vi "DetectorTest_MainV2.vi"() -> ()   [LabVIEW 2012]
uses:
  <vilib>/Analysis/NI_AALBase.lvlib
panel:
  out "Counter":i32
  out "NameList":string[](array[string])=["Diode_Open_3000", "Diode_Open_2000", "Diode_Open_1000", "Diode_Open_500", "Diode_Open_300", "Diode_Open_200", "Diode_Open_100", "Diode_Open_70", "Diode_Open_50", "Diode_Open_20", "Diode_Open_5_500", "Diode_Open_5_300", "Diode_Open_5_200", "Diode_Open_5_100", "Diode_Open_5_70", "Diode_Open_5_50", "Diode_Open_5_20", "Diode_Full_500", "Diode_Full_300", "Diode_Full_200", "Diode_Full_100", "Diode_Full_70", "Diode_Full_50", "Diode_Full_20", "Diode_Open_100_A", "Diode_Open_200_A", "QE_pad"]
  in  "Wafer Info Flash 2":T1={"Cell Name"="5500_130_05", "Package"="", "Coating"="", "LRC?"=enum."J2", "Comment"=""}
  in  "Parameters Flash 2":T2 {"Voc" format="%#_4g"; "Isc" format="%#_4g"; "FF" format="%#_4g"; "Imax" format="%#_4g"; "Vmax" format="%#_4g"; "Pmax" format="%#_4g"; "Itest" format="%#_4g"}
  in  "Wafer Info Flash":T1={"Cell Name"="Diode_Open_5_100", "Package"="", "Coating"="", "LRC?"=enum."J2", "Comment"=""}
  in  "Parameters Flash":T2={"Voc"=0.0, "Isc"=0.0, "FF"=0.0, "Vtest"=0.0, "Imax"=0.0, "Vmax"=0.0, "Pmax"=0.0, "Itest"=0.0, "Efficiency"=0.0, "P_in (W)"=0.0, "Irradiance (W/cm²)"=0.0, "Cell Area (cm²)"=12801.99006, "Number of AM1.5D Suns"=0.0, "Isotype Scalar"=0.0, "Equivalent 1 sun Jsc"=0.0} {"Voc" format="%#_4g"; "Isc" format="%#_4g"; "FF" format="%#_4g"; "Imax" format="%#_4g"; "Vmax" format="%#_4g"; "Pmax" format="%#_4g"; "Itest" format="%#_4g"}
  out "RawData file":path=path "C:/Users/Flash/Desktop/Data/Detector test data/A-3348-2-A_Diode_Open_5_100_20171205171726.csv"
  out "Fine Cell Clusters":T3(array[cluster])=[{"Cell Name"="Diode_Open_5_100", "X-coord"=56060.0, "Y-coord"=24330.0, "Area"=12801.99006, "Grid Shadowing"=0.0, "Xdim"=50.0, "Ydim"=50.0, "Mesa Area"=7853.981634}, {"Cell Name"="Diode_Open_5_100", "X-coord"=56060.0, "Y-coord"=14330.0, "Area"=12801.99006, "Grid Shadowing"=0.0, "Xdim"=50.0, "Ydim"=50.0, "Mesa Area"=7853.981634}, {"Cell Name"="Diode_Open_5_100", "X-coord"=-3940.0, "Y-coord"=4330.0, "Area"=12801.99006, "Grid Shadowing"=0.0, "Xdim"=50.0, "Ydim"=50.0, "Mesa Area"=7853.981634}, {"Cell Name"="Diode_Open_5_100", "X-coord"=-9540.0, "Y-coord"=10700.0, "Area"=12801.99006, "Grid Shadowing"=0.0, "Xdim"=50.0, "Ydim"=50.0, "Mesa Area"=7853.981634}, {"Cell Name"="Diode_Open_5_100", "X-coord"=46060.0, "Y-coord"=4330.0, "Area"=12801.99006, "Grid Shadowing"=0.0, "Xdim"=50.0, "Ydim"=50.0, "Mesa Area"=7853.981634}, {"Cell Name"="Diode_Open_5_100", "X-coord"=6060.0, "Y-coord"=-5670.0, "Area"=12801.99006, "Grid Shadowing"=0.0, "Xdim"=50.0, "Ydim"=50.0, "Mesa Area"=7853.981634}, {"Cell Name"="Diode_Open_5_100", "X-coord"=460.0, "Y-coord"=700.0, "Area"=12801.99006, "Grid Shadowing"=0.0, "Xdim"=50.0, "Ydim"=50.0, "Mesa Area"=7853.981634}, {"Cell Name"="Diode_Open_5_100", "X-coord"=16060.0, "Y-coord"=-5670.0, "Area"=12801.99006, "Grid Shadowing"=0.0, "Xdim"=50.0, "Ydim"=50.0, "Mesa Area"=7853.981634}, {"Cell Name"="Diode_Open_5_100", "X-coord"=26060.0, "Y-coord"=-5670.0, "Area"=12801.99006, "Grid Shadowing"=0.0, "Xdim"=50.0, "Ydim"=50.0, "Mesa Area"=7853.981634}, {"Cell Name"="Diode_Open_5_100", "X-coord"=30460.0, "Y-coord"=700.0, "Area"=12801.99006, "Grid Shadowing"=0.0, "Xdim"=50.0, "Ydim"=50.0, "Mesa Area"=7853.981634}]
  out "Selected Data":cluster{dbl[], dbl[]}={[nan, nan, nan, nan, nan, nan, nan, nan, nan, nan, nan, nan, nan, nan, nan, nan, nan, nan, nan, nan, nan, nan, nan, nan, nan, nan, nan, nan, nan, nan, nan, nan, nan, nan, nan, nan, nan, nan, nan, nan, nan, nan, nan, nan, nan, nan, nan, nan, nan, nan, nan, nan, nan, nan, nan, nan, nan, nan, nan, nan, nan, nan, nan, nan, nan, nan, nan, nan, nan, nan, nan, nan, nan, nan, nan, nan, nan, nan, nan, nan, nan, nan, nan, nan, nan, nan, nan, nan, nan, nan, nan, nan, nan, nan, nan, nan, nan, nan, nan, nan, nan, nan, nan, nan], [nan, nan, nan, nan, nan, nan, nan, nan, nan, nan, nan, nan, nan, nan, nan, nan, nan, nan, nan, nan, nan, nan, nan, nan, nan, nan, nan, nan, nan, nan, nan, nan, nan, nan, nan, nan, nan, nan, nan, nan, nan, nan, nan, nan, nan, nan, nan, nan, nan, nan, nan, nan, nan, nan, nan, nan, nan, nan, nan, nan, nan, nan, nan, nan, nan, nan, nan, nan, nan, nan, nan, nan, nan, nan, nan, nan, nan, nan, nan, nan, nan, nan, nan, nan, nan, nan, nan, nan, nan, nan, nan, nan, nan, nan, nan, nan, nan, nan, nan, nan, nan, nan, nan, nan]}
  in  "Test Results 2":T4
  in  "Session Info 2":T5={"V set"=-1.0, "I compliance"=0.001, "J set"=0.01, "I set"=0.0, "V compliance"=1.0, "Laser Power (mW)"=0.0, "TestID"=0, "Session Time"=timestamp(0 s since 1904-01-01), "Operator"="Radek"} {"V compliance" format="%#_6f"; "I compliance" format="%#_6e"}
  in  "Die Info 2":T6={"Device Name"="", "ActiveArea_um2"=3848.451, "MesaArea_um2"=3848.451, "x"=0.0, "y"=0.0}
  in  "Wafer Info 2":T7
  in  "Test Results":T4={"I meas"=-8.21153e-09, "V meas"=0.229564, "Time"=timestamp(3595368212.7604895 s since 1904-01-01)}
  in  "Session Info":T5={"V set"=-1.0, "I compliance"=0.001, "J set"=0.01, "I set"=1.5393804e-06, "V compliance"=1.0, "Laser Power (mW)"=0.0, "TestID"=289, "Session Time"=timestamp(3595367846.336531 s since 1904-01-01), "Operator"="pkawula"} {"V compliance" format="%#_6f"; "I compliance" format="%#_6e"}
  in  "Die Info":T6={"Device Name"="Diode_Open_5_100", "ActiveArea_um2"=12801.99006, "MesaArea_um2"=7853.981634, "x"=6060.0, "y"=44330.0}
  in  "Wafer Info":T7={"Wafer Name"="A-3348-2-A", "Scribe"="BG531-103", "Mask"="SL066", "Lot"="SJC_ENG_342_4"}
  in  "Name Array":string[](array[string])=["Wafer name", "Scribe", "Mask", "Lot", "Device name", "Active Area", "Mesa Area", "x", "y", "Imeas", "Vmeas", "Time", "Vset", "Icomp", "Jset", "Iset", "Vcomp", "Laser Power", "TestID", "SessionTime", "Operator", "Selected"]
  in  "TestID file":path=path "C:/Users/Flash/Desktop/LabVIEW/Detector IV/rawtest_log.csv"
  in  "update wafer":bool
  in  "Lot":string="SJC_ENG_342_4"
  in  "Laser Power (mW)":dbl
  in  "Device Name":string="Diode_Open_5_100"
  in  "Scribe":string="BG531-105"
  in  "MesaArea_um2":dbl=7853.981634
  out "Status":string="idle"
  out "error out":errorcluster
  in  "error in (no error)":errorcluster
  out "Manaul Plot 1":cluster{"V manual":dbl[], dbl[]}[](array[cluster])=[{"V manual"=[-1.5, -1.45128, -1.40256, -1.35385, -1.30513, -1.25641, -1.20769, -1.15897, -1.11026, -1.06154, -1.01282, -0.964103, -0.915385, -0.866667, -0.817949, -0.769231, -0.720513, -0.671795, -0.623077, -0.574359, -0.525641, -0.476923, -0.428205, -0.379487, -0.330769, -0.282051, -0.233333, -0.184615, -0.135897, -0.0871795, -0.0384615, 0.0102564, 0.0589744, 0.107692, 0.15641, 0.205128, 0.253846, 0.302564, 0.351282, 0.4], [0.000371182, 0.000368087, 0.000365666, 0.000361585, 0.000358777, 0.000355415, 0.000352273, 0.00034839, 0.000345122, 0.00034151, 0.00033751, 0.000332836, 0.000329855, 0.000326461, 0.000322528, 0.000317656, 0.000313266, 0.000310053, 0.000304697, 0.000300113, 0.00029575, 0.000290713, 0.000285749, 0.00028048, 0.000275303, 0.000269023, 0.000263057, 0.000256756, 0.000250067, 0.000242646, 0.000235352, 0.000226249, 0.000216807, 0.000205541, 0.000192231, 0.000174354, 0.000146988, 9.49448e-05, 1.32493e-05, 0.000227531]}, {"V manual"=[-1.0, nan, nan, nan, nan, nan, nan, nan, nan, nan, nan, nan, nan, nan, nan, nan, nan, nan, nan, nan, nan, nan, nan, nan, nan, nan, nan, nan, nan, nan, nan, nan, nan, nan, nan, nan, nan, nan, nan, nan], [0.0003364616, nan, nan, nan, nan, nan, nan, nan, nan, nan, nan, nan, nan, nan, nan, nan, nan, nan, nan, nan, nan, nan, nan, nan, nan, nan, nan, nan, nan, nan, nan, nan, nan, nan, nan, nan, nan, nan, nan, nan]}, {"V manual"=[0.369974, nan, nan, nan, nan, nan, nan, nan, nan, nan, nan, nan, nan, nan, nan, nan, nan, nan, nan, nan, nan, nan, nan, nan, nan, nan, nan, nan, nan, nan, nan, nan, nan, nan, nan, nan, nan, nan, nan, nan], [8.183848863e-05, nan, nan, nan, nan, nan, nan, nan, nan, nan, nan, nan, nan, nan, nan, nan, nan, nan, nan, nan, nan, nan, nan, nan, nan, nan, nan, nan, nan, nan, nan, nan, nan, nan, nan, nan, nan, nan, nan, nan]}]
  out "Manual Plot 0":cluster{"V manual":dbl[], "I manual":dbl[]}[](array[cluster])=[{"V manual"=[-1.5, -1.45128, -1.40256, -1.35385, -1.30513, -1.25641, -1.20769, -1.15897, -1.11026, -1.06154, -1.01282, -0.964103, -0.915385, -0.866667, -0.817949, -0.769231, -0.720513, -0.671795, -0.623077, -0.574359, -0.525641, -0.476923, -0.428205, -0.379487, -0.330769, -0.282051, -0.233333, -0.184615, -0.135897, -0.0871795, -0.0384615, 0.0102564, 0.0589744, 0.107692, 0.15641, 0.205128, 0.253846, 0.302564, 0.351282, 0.4], "I manual"=[-0.000371182, -0.000368087, -0.000365666, -0.000361585, -0.000358777, -0.000355415, -0.000352273, -0.00034839, -0.000345122, -0.00034151, -0.00033751, -0.000332836, -0.000329855, -0.000326461, -0.000322528, -0.000317656, -0.000313266, -0.000310053, -0.000304697, -0.000300113, -0.00029575, -0.000290713, -0.000285749, -0.00028048, -0.000275303, -0.000269023, -0.000263057, -0.000256756, -0.000250067, -0.000242646, -0.000235352, -0.000226249, -0.000216807, -0.000205541, -0.000192231, -0.000174354, -0.000146988, -9.49448e-05, 1.32493e-05, 0.000227531]}, {"V manual"=[-1.0, nan, nan, nan, nan, nan, nan, nan, nan, nan, nan, nan, nan, nan, nan, nan, nan, nan, nan, nan, nan, nan, nan, nan, nan, nan, nan, nan, nan, nan, nan, nan, nan, nan, nan, nan, nan, nan, nan, nan], "I manual"=[-0.0003364616, nan, nan, nan, nan, nan, nan, nan, nan, nan, nan, nan, nan, nan, nan, nan, nan, nan, nan, nan, nan, nan, nan, nan, nan, nan, nan, nan, nan, nan, nan, nan, nan, nan, nan, nan, nan, nan, nan, nan]}, {"V manual"=[0.369974, nan, nan, nan, nan, nan, nan, nan, nan, nan, nan, nan, nan, nan, nan, nan, nan, nan, nan, nan, nan, nan, nan, nan, nan, nan, nan, nan, nan, nan, nan, nan, nan, nan, nan, nan, nan, nan, nan, nan], "I manual"=[8.183848863e-05, nan, nan, nan, nan, nan, nan, nan, nan, nan, nan, nan, nan, nan, nan, nan, nan, nan, nan, nan, nan, nan, nan, nan, nan, nan, nan, nan, nan, nan, nan, nan, nan, nan, nan, nan, nan, nan, nan, nan]}]
  in  "Reset 1st die":bool
  in  "Sweep Settings":T8={"Channel"=enum."Channel A", "Vstart"=-2.0, "Vend"=0.5, "# of points"=30, "NPLC"=1.0, "I compliance"=0.001, "Delay ms"=500.0}
  in  "Reset xy":bool
  out "current y":i32
  out "current x":i32
  in  "sweep delay ms":dbl=500.0
  in  "I compliance":dbl=0.001
  in  "points":u16=40
  in  "V end":dbl=0.4
  in  "V start":dbl=-1.5
  in  "Repeat Vf":u32=1
  out "I set":dbl=7.853981633999999e-07
  in  "V compliance":dbl=1.0 format="%#_6f"
  in  "Vf delay ms":dbl=100.0
  in  "J set A/cm2":dbl=0.01
  in  "Repeat Id":u32=5
  in  "I compliance":dbl=0.001 format="%#_6e"
  in  "Id delay ms":dbl=500.0
  in  "V set":dbl=-1.0
  out "Vmeas Settings":T9={"Channel"=enum."Channel A", "Iset"=-1.0, "NPLC"=1.0, "V compliance"=0.001, "Repeat time"=3, "Delay ms"=500.0}
  out "Imeas Settings":T10={"Channel"=enum."Channel A", "Vset"=-1.0, "NPLC"=1.0, "I compliance"=0.001, "Repeat time"=3, "Delay ms"=500.0}
  out "Array of Cell Data Clusters":T11(array[cluster])=[{"Cell Name"="Diode_Open_5_100", "X-coord"=-13940.0, "Y-coord"=24330.0, "Area"=12801.99006, "Grid Shadowing"=0.0, "Ydim"=50.0, "Xdim"=50.0, "Meas Area"=7853.981634}, {"Cell Name"="Diode_Open_5_100", "X-coord"=-19540.0, "Y-coord"=30700.0, "Area"=12801.99006, "Grid Shadowing"=0.0, "Ydim"=50.0, "Xdim"=50.0, "Meas Area"=7853.981634}, {"Cell Name"="Diode_Open_5_100", "X-coord"=-3940.0, "Y-coord"=24330.0, "Area"=12801.99006, "Grid Shadowing"=0.0, "Ydim"=50.0, "Xdim"=50.0, "Meas Area"=7853.981634}, {"Cell Name"="Diode_Open_5_100", "X-coord"=-9540.0, "Y-coord"=30700.0, "Area"=12801.99006, "Grid Shadowing"=0.0, "Ydim"=50.0, "Xdim"=50.0, "Meas Area"=7853.981634}, {"Cell Name"="Diode_Open_5_100", "X-coord"=6060.0, "Y-coord"=24330.0, "Area"=12801.99006, "Grid Shadowing"=0.0, "Ydim"=50.0, "Xdim"=50.0, "Meas Area"=7853.981634}, {"Cell Name"="Diode_Open_5_100", "X-coord"=460.0, "Y-coord"=30700.0, "Area"=12801.99006, "Grid Shadowing"=0.0, "Ydim"=50.0, "Xdim"=50.0, "Meas Area"=7853.981634}, {"Cell Name"="Diode_Open_5_100", "X-coord"=16060.0, "Y-coord"=24330.0, "Area"=12801.99006, "Grid Shadowing"=0.0, "Ydim"=50.0, "Xdim"=50.0, "Meas Area"=7853.981634}, {"Cell Name"="Diode_Open_5_100", "X-coord"=10460.0, "Y-coord"=30700.0, "Area"=12801.99006, "Grid Shadowing"=0.0, "Ydim"=50.0, "Xdim"=50.0, "Meas Area"=7853.981634}, {"Cell Name"="Diode_Open_5_100", "X-coord"=26060.0, "Y-coord"=24330.0, "Area"=12801.99006, "Grid Shadowing"=0.0, "Ydim"=50.0, "Xdim"=50.0, "Meas Area"=7853.981634}, {"Cell Name"="Diode_Open_5_100", "X-coord"=20460.0, "Y-coord"=30700.0, "Area"=12801.99006, "Grid Shadowing"=0.0, "Ydim"=50.0, "Xdim"=50.0, "Meas Area"=7853.981634}, {"Cell Name"="Diode_Open_5_100", "X-coord"=36060.0, "Y-coord"=24330.0, "Area"=12801.99006, "Grid Shadowing"=0.0, "Ydim"=50.0, "Xdim"=50.0, "Meas Area"=7853.981634}, {"Cell Name"="Diode_Open_5_100", "X-coord"=30460.0, "Y-coord"=30700.0, "Area"=12801.99006, "Grid Shadowing"=0.0, "Ydim"=50.0, "Xdim"=50.0, "Meas Area"=7853.981634}, {"Cell Name"="Diode_Open_5_100", "X-coord"=46060.0, "Y-coord"=24330.0, "Area"=12801.99006, "Grid Shadowing"=0.0, "Ydim"=50.0, "Xdim"=50.0, "Meas Area"=7853.981634}, {"Cell Name"="Diode_Open_5_100", "X-coord"=40460.0, "Y-coord"=30700.0, "Area"=12801.99006, "Grid Shadowing"=0.0, "Ydim"=50.0, "Xdim"=50.0, "Meas Area"=7853.981634}, {"Cell Name"="Diode_Open_5_100", "X-coord"=56060.0, "Y-coord"=24330.0, "Area"=12801.99006, "Grid Shadowing"=0.0, "Ydim"=50.0, "Xdim"=50.0, "Meas Area"=7853.981634}, {"Cell Name"="Diode_Open_5_100", "X-coord"=50460.0, "Y-coord"=30700.0, "Area"=12801.99006, "Grid Shadowing"=0.0, "Ydim"=50.0, "Xdim"=50.0, "Meas Area"=7853.981634}, {"Cell Name"="Diode_Open_5_100", "X-coord"=-13940.0, "Y-coord"=14330.0, "Area"=12801.99006, "Grid Shadowing"=0.0, "Ydim"=50.0, "Xdim"=50.0, "Meas Area"=7853.981634}, {"Cell Name"="Diode_Open_5_100", "X-coord"=-19540.0, "Y-coord"=20700.0, "Area"=12801.99006, "Grid Shadowing"=0.0, "Ydim"=50.0, "Xdim"=50.0, "Meas Area"=7853.981634}, {"Cell Name"="Diode_Open_5_100", "X-coord"=-3940.0, "Y-coord"=14330.0, "Area"=12801.99006, "Grid Shadowing"=0.0, "Ydim"=50.0, "Xdim"=50.0, "Meas Area"=7853.981634}, {"Cell Name"="Diode_Open_5_100", "X-coord"=-9540.0, "Y-coord"=20700.0, "Area"=12801.99006, "Grid Shadowing"=0.0, "Ydim"=50.0, "Xdim"=50.0, "Meas Area"=7853.981634}, {"Cell Name"="Diode_Open_5_100", "X-coord"=16060.0, "Y-coord"=14330.0, "Area"=12801.99006, "Grid Shadowing"=0.0, "Ydim"=50.0, "Xdim"=50.0, "Meas Area"=7853.981634}, {"Cell Name"="Diode_Open_5_100", "X-coord"=10460.0, "Y-coord"=20700.0, "Area"=12801.99006, "Grid Shadowing"=0.0, "Ydim"=50.0, "Xdim"=50.0, "Meas Area"=7853.981634}, {"Cell Name"="Diode_Open_5_100", "X-coord"=26060.0, "Y-coord"=14330.0, "Area"=12801.99006, "Grid Shadowing"=0.0, "Ydim"=50.0, "Xdim"=50.0, "Meas Area"=7853.981634}, {"Cell Name"="Diode_Open_5_100", "X-coord"=20460.0, "Y-coord"=20700.0, "Area"=12801.99006, "Grid Shadowing"=0.0, "Ydim"=50.0, "Xdim"=50.0, "Meas Area"=7853.981634}, {"Cell Name"="Diode_Open_5_100", "X-coord"=46060.0, "Y-coord"=14330.0, "Area"=12801.99006, "Grid Shadowing"=0.0, "Ydim"=50.0, "Xdim"=50.0, "Meas Area"=7853.981634}, {"Cell Name"="Diode_Open_5_100", "X-coord"=40460.0, "Y-coord"=20700.0, "Area"=12801.99006, "Grid Shadowing"=0.0, "Ydim"=50.0, "Xdim"=50.0, "Meas Area"=7853.981634}, {"Cell Name"="Diode_Open_5_100", "X-coord"=56060.0, "Y-coord"=14330.0, "Area"=12801.99006, "Grid Shadowing"=0.0, "Ydim"=50.0, "Xdim"=50.0, "Meas Area"=7853.981634}, {"Cell Name"="Diode_Open_5_100", "X-coord"=50460.0, "Y-coord"=20700.0, "Area"=12801.99006, "Grid Shadowing"=0.0, "Ydim"=50.0, "Xdim"=50.0, "Meas Area"=7853.981634}, {"Cell Name"="Diode_Open_5_100", "X-coord"=-3940.0, "Y-coord"=4330.0, "Area"=12801.99006, "Grid Shadowing"=0.0, "Ydim"=50.0, "Xdim"=50.0, "Meas Area"=7853.981634}, {"Cell Name"="Diode_Open_5_100", "X-coord"=-9540.0, "Y-coord"=10700.0, "Area"=12801.99006, "Grid Shadowing"=0.0, "Ydim"=50.0, "Xdim"=50.0, "Meas Area"=7853.981634}, {"Cell Name"="Diode_Open_5_100", "X-coord"=6060.0, "Y-coord"=4330.0, "Area"=12801.99006, "Grid Shadowing"=0.0, "Ydim"=50.0, "Xdim"=50.0, "Meas Area"=7853.981634}, {"Cell Name"="Diode_Open_5_100", "X-coord"=460.0, "Y-coord"=10700.0, "Area"=12801.99006, "Grid Shadowing"=0.0, "Ydim"=50.0, "Xdim"=50.0, "Meas Area"=7853.981634}, {"Cell Name"="Diode_Open_5_100", "X-coord"=16060.0, "Y-coord"=4330.0, "Area"=12801.99006, "Grid Shadowing"=0.0, "Ydim"=50.0, "Xdim"=50.0, "Meas Area"=7853.981634}, {"Cell Name"="Diode_Open_5_100", "X-coord"=10460.0, "Y-coord"=10700.0, "Area"=12801.99006, "Grid Shadowing"=0.0, "Ydim"=50.0, "Xdim"=50.0, "Meas Area"=7853.981634}, {"Cell Name"="Diode_Open_5_100", "X-coord"=26060.0, "Y-coord"=4330.0, "Area"=12801.99006, "Grid Shadowing"=0.0, "Ydim"=50.0, "Xdim"=50.0, "Meas Area"=7853.981634}, {"Cell Name"="Diode_Open_5_100", "X-coord"=20460.0, "Y-coord"=10700.0, "Area"=12801.99006, "Grid Shadowing"=0.0, "Ydim"=50.0, "Xdim"=50.0, "Meas Area"=7853.981634}, {"Cell Name"="Diode_Open_5_100", "X-coord"=36060.0, "Y-coord"=4330.0, "Area"=12801.99006, "Grid Shadowing"=0.0, "Ydim"=50.0, "Xdim"=50.0, "Meas Area"=7853.981634}, {"Cell Name"="Diode_Open_5_100", "X-coord"=30460.0, "Y-coord"=10700.0, "Area"=12801.99006, "Grid Shadowing"=0.0, "Ydim"=50.0, "Xdim"=50.0, "Meas Area"=7853.981634}, {"Cell Name"="Diode_Open_5_100", "X-coord"=46060.0, "Y-coord"=4330.0, "Area"=12801.99006, "Grid Shadowing"=0.0, "Ydim"=50.0, "Xdim"=50.0, "Meas Area"=7853.981634}, {"Cell Name"="Diode_Open_5_100", "X-coord"=40460.0, "Y-coord"=10700.0, "Area"=12801.99006, "Grid Shadowing"=0.0, "Ydim"=50.0, "Xdim"=50.0, "Meas Area"=7853.981634}, {"Cell Name"="Diode_Open_5_100", "X-coord"=6060.0, "Y-coord"=-5670.0, "Area"=12801.99006, "Grid Shadowing"=0.0, "Ydim"=50.0, "Xdim"=50.0, "Meas Area"=7853.981634}, {"Cell Name"="Diode_Open_5_100", "X-coord"=460.0, "Y-coord"=700.0, "Area"=12801.99006, "Grid Shadowing"=0.0, "Ydim"=50.0, "Xdim"=50.0, "Meas Area"=7853.981634}, {"Cell Name"="Diode_Open_5_100", "X-coord"=16060.0, "Y-coord"=-5670.0, "Area"=12801.99006, "Grid Shadowing"=0.0, "Ydim"=50.0, "Xdim"=50.0, "Meas Area"=7853.981634}, {"Cell Name"="Diode_Open_5_100", "X-coord"=10460.0, "Y-coord"=700.0, "Area"=12801.99006, "Grid Shadowing"=0.0, "Ydim"=50.0, "Xdim"=50.0, "Meas Area"=7853.981634}, {"Cell Name"="Diode_Open_5_100", "X-coord"=26060.0, "Y-coord"=-5670.0, "Area"=12801.99006, "Grid Shadowing"=0.0, "Ydim"=50.0, "Xdim"=50.0, "Meas Area"=7853.981634}, {"Cell Name"="Diode_Open_5_100", "X-coord"=20460.0, "Y-coord"=700.0, "Area"=12801.99006, "Grid Shadowing"=0.0, "Ydim"=50.0, "Xdim"=50.0, "Meas Area"=7853.981634}, {"Cell Name"="Diode_Open_5_100", "X-coord"=36060.0, "Y-coord"=-5670.0, "Area"=12801.99006, "Grid Shadowing"=0.0, "Ydim"=50.0, "Xdim"=50.0, "Meas Area"=7853.981634}, {"Cell Name"="Diode_Open_5_100", "X-coord"=30460.0, "Y-coord"=700.0, "Area"=12801.99006, "Grid Shadowing"=0.0, "Ydim"=50.0, "Xdim"=50.0, "Meas Area"=7853.981634}, {"Cell Name"="Diode_Open_5_100", "X-coord"=6060.0, "Y-coord"=54330.0, "Area"=12801.99006, "Grid Shadowing"=0.0, "Ydim"=50.0, "Xdim"=50.0, "Meas Area"=7853.981634}, {"Cell Name"="Diode_Open_5_100", "X-coord"=460.0, "Y-coord"=60700.0, "Area"=12801.99006, "Grid Shadowing"=0.0, "Ydim"=50.0, "Xdim"=50.0, "Meas Area"=7853.981634}, {"Cell Name"="Diode_Open_5_100", "X-coord"=6060.0, "Y-coord"=64330.0, "Area"=12801.99006, "Grid Shadowing"=0.0, "Ydim"=50.0, "Xdim"=50.0, "Meas Area"=7853.981634}, {"Cell Name"="Diode_Open_5_100", "X-coord"=460.0, "Y-coord"=70700.0, "Area"=12801.99006, "Grid Shadowing"=0.0, "Ydim"=50.0, "Xdim"=50.0, "Meas Area"=7853.981634}, {"Cell Name"="Diode_Open_5_100", "X-coord"=16060.0, "Y-coord"=64330.0, "Area"=12801.99006, "Grid Shadowing"=0.0, "Ydim"=50.0, "Xdim"=50.0, "Meas Area"=7853.981634}, {"Cell Name"="Diode_Open_5_100", "X-coord"=10460.0, "Y-coord"=70700.0, "Area"=12801.99006, "Grid Shadowing"=0.0, "Ydim"=50.0, "Xdim"=50.0, "Meas Area"=7853.981634}, {"Cell Name"="Diode_Open_5_100", "X-coord"=26060.0, "Y-coord"=64330.0, "Area"=12801.99006, "Grid Shadowing"=0.0, "Ydim"=50.0, "Xdim"=50.0, "Meas Area"=7853.981634}, {"Cell Name"="Diode_Open_5_100", "X-coord"=20460.0, "Y-coord"=70700.0, "Area"=12801.99006, "Grid Shadowing"=0.0, "Ydim"=50.0, "Xdim"=50.0, "Meas Area"=7853.981634}, {"Cell Name"="Diode_Open_5_100", "X-coord"=36060.0, "Y-coord"=64330.0, "Area"=12801.99006, "Grid Shadowing"=0.0, "Ydim"=50.0, "Xdim"=50.0, "Meas Area"=7853.981634}, {"Cell Name"="Diode_Open_5_100", "X-coord"=30460.0, "Y-coord"=70700.0, "Area"=12801.99006, "Grid Shadowing"=0.0, "Ydim"=50.0, "Xdim"=50.0, "Meas Area"=7853.981634}, {"Cell Name"="Diode_Open_5_100", "X-coord"=-3940.0, "Y-coord"=54330.0, "Area"=12801.99006, "Grid Shadowing"=0.0, "Ydim"=50.0, "Xdim"=50.0, "Meas Area"=7853.981634}, {"Cell Name"="Diode_Open_5_100", "X-coord"=-9540.0, "Y-coord"=60700.0, "Area"=12801.99006, "Grid Shadowing"=0.0, "Ydim"=50.0, "Xdim"=50.0, "Meas Area"=7853.981634}, {"Cell Name"="Diode_Open_5_100", "X-coord"=16060.0, "Y-coord"=54330.0, "Area"=12801.99006, "Grid Shadowing"=0.0, "Ydim"=50.0, "Xdim"=50.0, "Meas Area"=7853.981634}, {"Cell Name"="Diode_Open_5_100", "X-coord"=10460.0, "Y-coord"=60700.0, "Area"=12801.99006, "Grid Shadowing"=0.0, "Ydim"=50.0, "Xdim"=50.0, "Meas Area"=7853.981634}, {"Cell Name"="Diode_Open_5_100", "X-coord"=26060.0, "Y-coord"=54330.0, "Area"=12801.99006, "Grid Shadowing"=0.0, "Ydim"=50.0, "Xdim"=50.0, "Meas Area"=7853.981634}, {"Cell Name"="Diode_Open_5_100", "X-coord"=20460.0, "Y-coord"=60700.0, "Area"=12801.99006, "Grid Shadowing"=0.0, "Ydim"=50.0, "Xdim"=50.0, "Meas Area"=7853.981634}, {"Cell Name"="Diode_Open_5_100", "X-coord"=36060.0, "Y-coord"=54330.0, "Area"=12801.99006, "Grid Shadowing"=0.0, "Ydim"=50.0, "Xdim"=50.0, "Meas Area"=7853.981634}, {"Cell Name"="Diode_Open_5_100", "X-coord"=30460.0, "Y-coord"=60700.0, "Area"=12801.99006, "Grid Shadowing"=0.0, "Ydim"=50.0, "Xdim"=50.0, "Meas Area"=7853.981634}, {"Cell Name"="Diode_Open_5_100", "X-coord"=46060.0, "Y-coord"=54330.0, "Area"=12801.99006, "Grid Shadowing"=0.0, "Ydim"=50.0, "Xdim"=50.0, "Meas Area"=7853.981634}, {"Cell Name"="Diode_Open_5_100", "X-coord"=40460.0, "Y-coord"=60700.0, "Area"=12801.99006, "Grid Shadowing"=0.0, "Ydim"=50.0, "Xdim"=50.0, "Meas Area"=7853.981634}, {"Cell Name"="Diode_Open_5_100", "X-coord"=-13940.0, "Y-coord"=44330.0, "Area"=12801.99006, "Grid Shadowing"=0.0, "Ydim"=50.0, "Xdim"=50.0, "Meas Area"=7853.981634}, {"Cell Name"="Diode_Open_5_100", "X-coord"=-19540.0, "Y-coord"=50700.0, "Area"=12801.99006, "Grid Shadowing"=0.0, "Ydim"=50.0, "Xdim"=50.0, "Meas Area"=7853.981634}, {"Cell Name"="Diode_Open_5_100", "X-coord"=-3940.0, "Y-coord"=44330.0, "Area"=12801.99006, "Grid Shadowing"=0.0, "Ydim"=50.0, "Xdim"=50.0, "Meas Area"=7853.981634}, {"Cell Name"="Diode_Open_5_100", "X-coord"=-9540.0, "Y-coord"=50700.0, "Area"=12801.99006, "Grid Shadowing"=0.0, "Ydim"=50.0, "Xdim"=50.0, "Meas Area"=7853.981634}, {"Cell Name"="Diode_Open_5_100", "X-coord"=56060.0, "Y-coord"=34330.0, "Area"=12801.99006, "Grid Shadowing"=0.0, "Ydim"=50.0, "Xdim"=50.0, "Meas Area"=7853.981634}, {"Cell Name"="Diode_Open_5_100", "X-coord"=50460.0, "Y-coord"=40700.0, "Area"=12801.99006, "Grid Shadowing"=0.0, "Ydim"=50.0, "Xdim"=50.0, "Meas Area"=7853.981634}, {"Cell Name"="Diode_Open_5_100", "X-coord"=46060.0, "Y-coord"=34330.0, "Area"=12801.99006, "Grid Shadowing"=0.0, "Ydim"=50.0, "Xdim"=50.0, "Meas Area"=7853.981634}, {"Cell Name"="Diode_Open_5_100", "X-coord"=40460.0, "Y-coord"=40700.0, "Area"=12801.99006, "Grid Shadowing"=0.0, "Ydim"=50.0, "Xdim"=50.0, "Meas Area"=7853.981634}, {"Cell Name"="Diode_Open_5_100", "X-coord"=36060.0, "Y-coord"=34330.0, "Area"=12801.99006, "Grid Shadowing"=0.0, "Ydim"=50.0, "Xdim"=50.0, "Meas Area"=7853.981634}, {"Cell Name"="Diode_Open_5_100", "X-coord"=30460.0, "Y-coord"=40700.0, "Area"=12801.99006, "Grid Shadowing"=0.0, "Ydim"=50.0, "Xdim"=50.0, "Meas Area"=7853.981634}, {"Cell Name"="Diode_Open_5_100", "X-coord"=26060.0, "Y-coord"=34330.0, "Area"=12801.99006, "Grid Shadowing"=0.0, "Ydim"=50.0, "Xdim"=50.0, "Meas Area"=7853.981634}, {"Cell Name"="Diode_Open_5_100", "X-coord"=20460.0, "Y-coord"=40700.0, "Area"=12801.99006, "Grid Shadowing"=0.0, "Ydim"=50.0, "Xdim"=50.0, "Meas Area"=7853.981634}, {"Cell Name"="Diode_Open_5_100", "X-coord"=16060.0, "Y-coord"=34330.0, "Area"=12801.99006, "Grid Shadowing"=0.0, "Ydim"=50.0, "Xdim"=50.0, "Meas Area"=7853.981634}, {"Cell Name"="Diode_Open_5_100", "X-coord"=10460.0, "Y-coord"=40700.0, "Area"=12801.99006, "Grid Shadowing"=0.0, "Ydim"=50.0, "Xdim"=50.0, "Meas Area"=7853.981634}, {"Cell Name"="Diode_Open_5_100", "X-coord"=6060.0, "Y-coord"=34330.0, "Area"=12801.99006, "Grid Shadowing"=0.0, "Ydim"=50.0, "Xdim"=50.0, "Meas Area"=7853.981634}, {"Cell Name"="Diode_Open_5_100", "X-coord"=460.0, "Y-coord"=40700.0, "Area"=12801.99006, "Grid Shadowing"=0.0, "Ydim"=50.0, "Xdim"=50.0, "Meas Area"=7853.981634}, {"Cell Name"="Diode_Open_5_100", "X-coord"=-3940.0, "Y-coord"=34330.0, "Area"=12801.99006, "Grid Shadowing"=0.0, "Ydim"=50.0, "Xdim"=50.0, "Meas Area"=7853.981634}, {"Cell Name"="Diode_Open_5_100", "X-coord"=-9540.0, "Y-coord"=40700.0, "Area"=12801.99006, "Grid Shadowing"=0.0, "Ydim"=50.0, "Xdim"=50.0, "Meas Area"=7853.981634}, {"Cell Name"="Diode_Open_5_100", "X-coord"=-13940.0, "Y-coord"=34330.0, "Area"=12801.99006, "Grid Shadowing"=0.0, "Ydim"=50.0, "Xdim"=50.0, "Meas Area"=7853.981634}, {"Cell Name"="Diode_Open_5_100", "X-coord"=-19540.0, "Y-coord"=40700.0, "Area"=12801.99006, "Grid Shadowing"=0.0, "Ydim"=50.0, "Xdim"=50.0, "Meas Area"=7853.981634}, {"Cell Name"="Diode_Open_5_100", "X-coord"=56060.0, "Y-coord"=44330.0, "Area"=12801.99006, "Grid Shadowing"=0.0, "Ydim"=50.0, "Xdim"=50.0, "Meas Area"=7853.981634}, {"Cell Name"="Diode_Open_5_100", "X-coord"=50460.0, "Y-coord"=50700.0, "Area"=12801.99006, "Grid Shadowing"=0.0, "Ydim"=50.0, "Xdim"=50.0, "Meas Area"=7853.981634}, {"Cell Name"="Diode_Open_5_100", "X-coord"=46060.0, "Y-coord"=44330.0, "Area"=12801.99006, "Grid Shadowing"=0.0, "Ydim"=50.0, "Xdim"=50.0, "Meas Area"=7853.981634}, {"Cell Name"="Diode_Open_5_100", "X-coord"=40460.0, "Y-coord"=50700.0, "Area"=12801.99006, "Grid Shadowing"=0.0, "Ydim"=50.0, "Xdim"=50.0, "Meas Area"=7853.981634}, {"Cell Name"="Diode_Open_5_100", "X-coord"=26060.0, "Y-coord"=44330.0, "Area"=12801.99006, "Grid Shadowing"=0.0, "Ydim"=50.0, "Xdim"=50.0, "Meas Area"=7853.981634}, {"Cell Name"="Diode_Open_5_100", "X-coord"=20460.0, "Y-coord"=50700.0, "Area"=12801.99006, "Grid Shadowing"=0.0, "Ydim"=50.0, "Xdim"=50.0, "Meas Area"=7853.981634}, {"Cell Name"="Diode_Open_5_100", "X-coord"=16060.0, "Y-coord"=44330.0, "Area"=12801.99006, "Grid Shadowing"=0.0, "Ydim"=50.0, "Xdim"=50.0, "Meas Area"=7853.981634}, {"Cell Name"="Diode_Open_5_100", "X-coord"=10460.0, "Y-coord"=50700.0, "Area"=12801.99006, "Grid Shadowing"=0.0, "Ydim"=50.0, "Xdim"=50.0, "Meas Area"=7853.981634}, {"Cell Name"="Diode_Open_5_100", "X-coord"=30460.0, "Y-coord"=20700.0, "Area"=12801.99006, "Grid Shadowing"=0.0, "Ydim"=50.0, "Xdim"=50.0, "Meas Area"=7853.981634}, {"Cell Name"="Diode_Open_5_100", "X-coord"=36060.0, "Y-coord"=14330.0, "Area"=12801.99006, "Grid Shadowing"=0.0, "Ydim"=50.0, "Xdim"=50.0, "Meas Area"=7853.981634}, {"Cell Name"="Diode_Open_5_100", "X-coord"=460.0, "Y-coord"=20700.0, "Area"=12801.99006, "Grid Shadowing"=0.0, "Ydim"=50.0, "Xdim"=50.0, "Meas Area"=7853.981634}, {"Cell Name"="Diode_Open_5_100", "X-coord"=6060.0, "Y-coord"=14330.0, "Area"=12801.99006, "Grid Shadowing"=0.0, "Ydim"=50.0, "Xdim"=50.0, "Meas Area"=7853.981634}, {"Cell Name"="Diode_Open_5_100", "X-coord"=30460.0, "Y-coord"=50700.0, "Area"=12801.99006, "Grid Shadowing"=0.0, "Ydim"=50.0, "Xdim"=50.0, "Meas Area"=7853.981634}, {"Cell Name"="Diode_Open_5_100", "X-coord"=36060.0, "Y-coord"=44330.0, "Area"=12801.99006, "Grid Shadowing"=0.0, "Ydim"=50.0, "Xdim"=50.0, "Meas Area"=7853.981634}, {"Cell Name"="Diode_Open_5_100", "X-coord"=460.0, "Y-coord"=50700.0, "Area"=12801.99006, "Grid Shadowing"=0.0, "Ydim"=50.0, "Xdim"=50.0, "Meas Area"=7853.981634}, {"Cell Name"="Diode_Open_5_100", "X-coord"=6060.0, "Y-coord"=44330.0, "Area"=12801.99006, "Grid Shadowing"=0.0, "Ydim"=50.0, "Xdim"=50.0, "Meas Area"=7853.981634}]
  in  "stop":bool
  in  "ActiveArea_um2":dbl=12801.99006
  in  "NPLC":dbl=1.0
  in  "Operator":string(combo)="pkawula"
  in  "Mask":string="SL066"
  in  "Wafer Name":string="A-3348-3-A"
  in  "Tab Control":T12(tab)
  in  "Start auto":bool
  in  "Clear List":bool
  in  "Refresh Device":bool
  in  "Mask Name":string="SL066"
  in  "Remove from List":bool
  in  "Add to list":bool
  in  "Available Device Name":string(combo)="Diode_Open_200_A"
  in  "Test List":i32(listbox)=-1
  in  "Mask File all":path=path "C:/Users/Flash/Desktop/Mask Files/SL066 Detector/SL066_mask_map_file_V3_align on D3000.csv"
  in  "Manual_Test":bool
  in  "Manual IV settting":enum32{"Linear plot", "Log plot"}(radio)
  out "Vmeas manual":dbl=0.369974
  out "Imeas manual":dbl=-0.0003364616
  out "Iarray manual":dbl[](array[numeric])=[-0.000371182, -0.000368087, -0.000365666, -0.000361585, -0.000358777, -0.000355415, -0.000352273, -0.00034839, -0.000345122, -0.00034151, -0.00033751, -0.000332836, -0.000329855, -0.000326461, -0.000322528, -0.000317656, -0.000313266, -0.000310053, -0.000304697, -0.000300113, -0.00029575, -0.000290713, -0.000285749, -0.00028048, -0.000275303, -0.000269023, -0.000263057, -0.000256756, -0.000250067, -0.000242646, -0.000235352, -0.000226249, -0.000216807, -0.000205541, -0.000192231, -0.000174354, -0.000146988, -9.49448e-05, 1.32493e-05, 0.000227531]
  out "Varray manual":dbl[](array[numeric])=[-1.5, -1.45128, -1.40256, -1.35385, -1.30513, -1.25641, -1.20769, -1.15897, -1.11026, -1.06154, -1.01282, -0.964103, -0.915385, -0.866667, -0.817949, -0.769231, -0.720513, -0.671795, -0.623077, -0.574359, -0.525641, -0.476923, -0.428205, -0.379487, -0.330769, -0.282051, -0.233333, -0.184615, -0.135897, -0.0871795, -0.0384615, 0.0102564, 0.0589744, 0.107692, 0.15641, 0.205128, 0.253846, 0.302564, 0.351282, 0.4]
  out "y target":i32=28070
  out "x target":i32=-15300
  in  "Die Number":u16(ring) items=["0", "1", "2", "3", "4", "5", "6", "7", "8", "9", "10", "11", "12", "13", "14", "15", "16", "17", "18", "19", "20", "21", "22", "23", "24", "25", "26", "27", "28", "29", "30", "31", "32", "33", "34", "35", "36", "37", "38", "39", "40", "41", "42", "43", "44", "45", "46", "47", "48", "49", "50", "51", "52", "53", "54", "55", "56", "57", "58", "59", "60", "61", "62", "63", "64", "65", "66", "67", "68", "69", "70", "71", "72", "73", "74", "75", "76", "77", "78", "79", "80", "81", "82", "83", "84", "85", "86", "87", "88", "89", "90", "91", "92", "93", "94", "95", "96", "97", "98", "99", "100", "101", "102", "103"]
  in  "load file":bool
  in  "Move to":bool
  in  "Mask File Manual":path=path "C:/Users/Flash/Desktop/Mask Files/SL066 Detector/SL066_mask_map_file_V3_align on D3000_Diode_Open_1000.csv"
  out "Manual IV":cluster{"V manual":dbl[], "I manual":dbl[]}[](graph)=[{"V manual"=[-1.5, -1.45128, -1.40256, -1.35385, -1.30513, -1.25641, -1.20769, -1.15897, -1.11026, -1.06154, -1.01282, -0.964103, -0.915385, -0.866667, -0.817949, -0.769231, -0.720513, -0.671795, -0.623077, -0.574359, -0.525641, -0.476923, -0.428205, -0.379487, -0.330769, -0.282051, -0.233333, -0.184615, -0.135897, -0.0871795, -0.0384615, 0.0102564, 0.0589744, 0.107692, 0.15641, 0.205128, 0.253846, 0.302564, 0.351282, 0.4], "I manual"=[-0.000371182, -0.000368087, -0.000365666, -0.000361585, -0.000358777, -0.000355415, -0.000352273, -0.00034839, -0.000345122, -0.00034151, -0.00033751, -0.000332836, -0.000329855, -0.000326461, -0.000322528, -0.000317656, -0.000313266, -0.000310053, -0.000304697, -0.000300113, -0.00029575, -0.000290713, -0.000285749, -0.00028048, -0.000275303, -0.000269023, -0.000263057, -0.000256756, -0.000250067, -0.000242646, -0.000235352, -0.000226249, -0.000216807, -0.000205541, -0.000192231, -0.000174354, -0.000146988, -9.49448e-05, 1.32493e-05, 0.000227531]}, {"V manual"=[-1.0, nan, nan, nan, nan, nan, nan, nan, nan, nan, nan, nan, nan, nan, nan, nan, nan, nan, nan, nan, nan, nan, nan, nan, nan, nan, nan, nan, nan, nan, nan, nan, nan, nan, nan, nan, nan, nan, nan, nan], "I manual"=[-0.0003364616, nan, nan, nan, nan, nan, nan, nan, nan, nan, nan, nan, nan, nan, nan, nan, nan, nan, nan, nan, nan, nan, nan, nan, nan, nan, nan, nan, nan, nan, nan, nan, nan, nan, nan, nan, nan, nan, nan, nan]}, {"V manual"=[0.369974, nan, nan, nan, nan, nan, nan, nan, nan, nan, nan, nan, nan, nan, nan, nan, nan, nan, nan, nan, nan, nan, nan, nan, nan, nan, nan, nan, nan, nan, nan, nan, nan, nan, nan, nan, nan, nan, nan, nan], "I manual"=[8.183848863e-05, nan, nan, nan, nan, nan, nan, nan, nan, nan, nan, nan, nan, nan, nan, nan, nan, nan, nan, nan, nan, nan, nan, nan, nan, nan, nan, nan, nan, nan, nan, nan, nan, nan, nan, nan, nan, nan, nan, nan]}]
  in  "Load raw":bool
  in  "Select":bool
  in  "Number Select":u16=10
  in  "Vmax":dbl=0.95
  in  "Vmin":dbl=0.05
  out "Test FileName":string="A-3348-2-A_Diode_Open_5_100_20171205171726.csv"
  out "RawTest ID":u32=289
  out "Progress":u8(slide)=99 scale=0.0..100.0
  out "Current Device":u32=104
  out "Total Device":u32=104
  out "V meas":dbl[](array[numeric])=[0.233008, 0.99988, 0.230081, 0.231856, 0.222896, 0.227718, 0.220368, 0.221624, 0.223083, 0.225844, 0.224788, 0.226016, 0.230367, 0.226863, 0.236152, 0.999885, 0.236278, 0.231894, 0.227969, 0.231092, 0.223719, 0.223157, 0.221075, 0.223088, 0.229423, 0.227845, 0.234104, 0.999884, 0.236984, 0.234402, 0.229175, 0.22777, 0.221645, 0.226168, 0.222958, 0.221157, 0.226097, 0.22608, 0.22911, 0.227312, 0.233594, 0.239497, 0.228026, 0.226055, 0.22758, 0.222034, 0.225611, 0.229698, 0.235983, 0.999873, 0.999878, 0.999876, 0.999884, 0.99988, 0.999881, 0.999878, 0.999876, 0.999876, 0.242386, 0.999877, 0.232405, 0.999877, 0.232378, 0.999881, 0.235204, 0.999878, 0.999878, 0.999878, 0.240209, 0.23837, 0.999879, 0.241394, 0.999882, 0.999877, 0.232764, 0.231476, 0.227194, 0.228614, 0.227446, 0.225845, 0.222835, 0.226481, 0.225718, 0.229356, 0.232511, 0.999874, 0.999878, 0.999879, 0.511839, 0.999881, 0.236876, 0.237455, 0.224476, 0.236416, 0.222221, 0.230631, 0.225214, 0.22589, 0.226556, 0.226418, 0.234927, 0.233388, 0.237265, 0.229564]
  out "I meas":dbl[](array[numeric])=[-1.791366e-08, -1.1957407999999998e-10, -8.510296e-09, -1.1848348e-08, -1.0634712e-08, -7.94538e-09, -1.0664641999999998e-08, -1.5484518e-08, -1.2807029999999998e-08, -1.2872500000000002e-08, -8.70304e-09, -1.0948554000000001e-08, -6.430202000000001e-09, -8.940911999999999e-09, -4.269804e-09, -2.3908200000000002e-09, -6.1184e-09, -7.475178e-09, -9.294318e-09, -1.0505516000000001e-08, -7.3206440000000005e-09, -8.520726e-09, -8.80908e-09, -1.0621755999999999e-08, -6.43336e-09, -8.429852e-09, -5.041916000000001e-09, -1.9718416e-10, -4.6682759999999995e-09, -5.138274e-09, -6.394414e-09, -7.840453999999999e-09, -8.213534e-09, -8.437916e-09, -8.39969e-09, -1.0195582e-08, -5.942146e-09, -7.641714e-09, -4.799278e-09, -6.2362860000000006e-09, -4.420012e-09, -3.2603080000000005e-09, -5.559286e-09, -5.7098779999999995e-09, -5.365526e-09, -7.813004e-09, -6.011059999999999e-09, -5.480968e-09, -1.035395e-08, 7.317542e-11, -6.2418100000000004e-12, 2.8383740000000004e-11, 3.794192e-11, 4.911428e-12, 2.923012e-11, 2.809286e-11, 3.036024e-11, -1.6028400000000002e-10, -9.937287999999999e-09, 4.2383680000000005e-11, -1.1358554000000001e-08, 3.9725299999999996e-11, -1.0078494000000001e-08, 6.30498e-11, -7.550982e-09, 8.784526e-11, -5.557216e-10, -9.84718e-11, -7.308986e-09, -1.3814348000000002e-08, 7.365464000000002e-11, -8.052186000000001e-09, -1.1067396e-11, -2.554022e-09, -7.325092e-09, -7.05232e-09, -9.755659999999999e-09, -1.1196856000000001e-08, -1.4346882000000001e-08, -1.4860736000000002e-08, -1.5036204e-08, -1.3369388e-08, -1.0021694e-08, -9.621842e-09, -8.068194e-09, 5.4979339999999994e-11, 5.7530419999999994e-12, -3.246182e-09, -4.980356000000001e-09, -2.7533859999999997e-09, -6.70936e-09, -6.9177280000000005e-09, -1.4554624e-08, -1.4164096000000001e-08, -1.6854384e-08, -1.380222e-08, -7.668758e-09, -5.926224e-09, -1.1557444000000001e-08, -7.354524000000001e-09, -8.160112000000001e-09, -9.152704000000001e-09, -1.1161659999999998e-08, -8.21153e-09]
  in  "RawData Save Path":path=path "C:/Users/Flash/Desktop/Data/Detector test data"
  in  "StartRaw":bool
  out "Vforward hist":T13(graph)={"X Values"=[0.25934385, 0.33729555, 0.41524725, 0.49319895, 0.57115065, 0.64910235, 0.72705405, 0.80500575, 0.88295745, 0.96090915], "Histogram: h(x)"=[78, 0, 0, 1, 0, 0, 0, 0, 0, 25]}
  out "Idark hist":T13(graph)={"X Values"=[-1.7013584737e-08, -1.5213434211e-08, -1.3413283685000001e-08, -1.1613133159000001e-08, -9.812982633000001e-09, -8.012832107e-09, -6.212681581000001e-09, -4.4125310550000005e-09, -2.6123805290000004e-09, -8.12230003e-10], "Histogram: h(x)"=[2, 5, 6, 6, 14, 23, 15, 7, 5, 21]}
  in  "Mask File Raw":path=path "C:/Users/Flash/Desktop/Mask Files/SL066 Detector/SL066_mask_map_file_V3_align on D3000_Diode_Open_5_100.csv"
  out "Spec Plot":cluster{"V meas":dbl[], "I meas":dbl[]}[](graph)=[{"V meas"=[0.233008, 0.99988, 0.230081, 0.231856, 0.222896, 0.227718, 0.220368, 0.221624, 0.223083, 0.225844, 0.224788, 0.226016, 0.230367, 0.226863, 0.236152, 0.999885, 0.236278, 0.231894, 0.227969, 0.231092, 0.223719, 0.223157, 0.221075, 0.223088, 0.229423, 0.227845, 0.234104, 0.999884, 0.236984, 0.234402, 0.229175, 0.22777, 0.221645, 0.226168, 0.222958, 0.221157, 0.226097, 0.22608, 0.22911, 0.227312, 0.233594, 0.239497, 0.228026, 0.226055, 0.22758, 0.222034, 0.225611, 0.229698, 0.235983, 0.999873, 0.999878, 0.999876, 0.999884, 0.99988, 0.999881, 0.999878, 0.999876, 0.999876, 0.242386, 0.999877, 0.232405, 0.999877, 0.232378, 0.999881, 0.235204, 0.999878, 0.999878, 0.999878, 0.240209, 0.23837, 0.999879, 0.241394, 0.999882, 0.999877, 0.232764, 0.231476, 0.227194, 0.228614, 0.227446, 0.225845, 0.222835, 0.226481, 0.225718, 0.229356, 0.232511, 0.999874, 0.999878, 0.999879, 0.511839, 0.999881, 0.236876, 0.237455, 0.224476, 0.236416, 0.222221, 0.230631, 0.225214, 0.22589, 0.226556, 0.226418, 0.234927, 0.233388, 0.237265, 0.229564], "I meas"=[-1.791366e-08, -1.1957407999999998e-10, -8.510296e-09, -1.1848348e-08, -1.0634712e-08, -7.94538e-09, -1.0664641999999998e-08, -1.5484518e-08, -1.2807029999999998e-08, -1.2872500000000002e-08, -8.70304e-09, -1.0948554000000001e-08, -6.430202000000001e-09, -8.940911999999999e-09, -4.269804e-09, -2.3908200000000002e-09, -6.1184e-09, -7.475178e-09, -9.294318e-09, -1.0505516000000001e-08, -7.3206440000000005e-09, -8.520726e-09, -8.80908e-09, -1.0621755999999999e-08, -6.43336e-09, -8.429852e-09, -5.041916000000001e-09, -1.9718416e-10, -4.6682759999999995e-09, -5.138274e-09, -6.394414e-09, -7.840453999999999e-09, -8.213534e-09, -8.437916e-09, -8.39969e-09, -1.0195582e-08, -5.942146e-09, -7.641714e-09, -4.799278e-09, -6.2362860000000006e-09, -4.420012e-09, -3.2603080000000005e-09, -5.559286e-09, -5.7098779999999995e-09, -5.365526e-09, -7.813004e-09, -6.011059999999999e-09, -5.480968e-09, -1.035395e-08, 7.317542e-11, -6.2418100000000004e-12, 2.8383740000000004e-11, 3.794192e-11, 4.911428e-12, 2.923012e-11, 2.809286e-11, 3.036024e-11, -1.6028400000000002e-10, -9.937287999999999e-09, 4.2383680000000005e-11, -1.1358554000000001e-08, 3.9725299999999996e-11, -1.0078494000000001e-08, 6.30498e-11, -7.550982e-09, 8.784526e-11, -5.557216e-10, -9.84718e-11, -7.308986e-09, -1.3814348000000002e-08, 7.365464000000002e-11, -8.052186000000001e-09, -1.1067396e-11, -2.554022e-09, -7.325092e-09, -7.05232e-09, -9.755659999999999e-09, -1.1196856000000001e-08, -1.4346882000000001e-08, -1.4860736000000002e-08, -1.5036204e-08, -1.3369388e-08, -1.0021694e-08, -9.621842e-09, -8.068194e-09, 5.4979339999999994e-11, 5.7530419999999994e-12, -3.246182e-09, -4.980356000000001e-09, -2.7533859999999997e-09, -6.70936e-09, -6.9177280000000005e-09, -1.4554624e-08, -1.4164096000000001e-08, -1.6854384e-08, -1.380222e-08, -7.668758e-09, -5.926224e-09, -1.1557444000000001e-08, -7.354524000000001e-09, -8.160112000000001e-09, -9.152704000000001e-09, -1.1161659999999998e-08, -8.21153e-09]}, {"V meas"=[0.236152, 0.234104, 0.236984, 0.234402, 0.22911, 0.233594, 0.239497, 0.228026, 0.22758, 0.229698, nan, nan, nan, nan, nan, nan, nan, nan, nan, nan, nan, nan, nan, nan, nan, nan, nan, nan, nan, nan, nan, nan, nan, nan, nan, nan, nan, nan, nan, nan, nan, nan, nan, nan, nan, nan, nan, nan, nan, nan, nan, nan, nan, nan, nan, nan, nan, nan, nan, nan, nan, nan, nan, nan, nan, nan, nan, nan, nan, nan, nan, nan, nan, nan, nan, nan, nan, nan, nan, nan, nan, nan, nan, nan, nan, nan, nan, nan, nan, nan, nan, nan, nan, nan, nan, nan, nan, nan, nan, nan, nan, nan, nan, nan], "I meas"=[-4.269804e-09, -5.041916000000001e-09, -4.6682759999999995e-09, -5.138274e-09, -4.799278e-09, -4.420012e-09, -3.2603080000000005e-09, -5.559286e-09, -5.365526e-09, -5.480968e-09, nan, nan, nan, nan, nan, nan, nan, nan, nan, nan, nan, nan, nan, nan, nan, nan, nan, nan, nan, nan, nan, nan, nan, nan, nan, nan, nan, nan, nan, nan, nan, nan, nan, nan, nan, nan, nan, nan, nan, nan, nan, nan, nan, nan, nan, nan, nan, nan, nan, nan, nan, nan, nan, nan, nan, nan, nan, nan, nan, nan, nan, nan, nan, nan, nan, nan, nan, nan, nan, nan, nan, nan, nan, nan, nan, nan, nan, nan, nan, nan, nan, nan, nan, nan, nan, nan, nan, nan, nan, nan, nan, nan, nan, nan]}]
  in  "FineTest save path":path=path "C:/Users/Flash/Desktop/Data/Detector test data/IV"
  out "I fine":dbl[](array[numeric])=[-1.52182e-05, -1.47166e-05, -1.48638e-05, -1.4948e-05, -1.49634e-05, -1.49403e-05, -1.48575e-05, -1.48749e-05, -1.47754e-05, -1.47251e-05, -1.46559e-05, -1.45851e-05, -1.45028e-05, -1.43852e-05, -1.42468e-05, -1.41684e-05, -1.40308e-05, -1.39364e-05, -1.37397e-05, -1.35679e-05, -1.3482e-05, -1.32093e-05, -1.2996e-05, -1.28281e-05, -1.25632e-05, -1.23417e-05, -1.20643e-05, -1.17371e-05, -1.14516e-05, -1.10657e-05, -1.06617e-05, -1.02025e-05, -9.26216e-06, -9.00798e-06, -8.21814e-06, -7.12779e-06, -5.50195e-06, -2.50105e-06, 4.02524e-06, 2.01571e-05]
  out "V fine":dbl[](array[numeric])=[-1.5, -1.45128, -1.40256, -1.35385, -1.30513, -1.25641, -1.20769, -1.15897, -1.11026, -1.06154, -1.01282, -0.964103, -0.915385, -0.866667, -0.817949, -0.769231, -0.720513, -0.671795, -0.623077, -0.574359, -0.525641, -0.476923, -0.428205, -0.379487, -0.330769, -0.282051, -0.233333, -0.184615, -0.135897, -0.0871795, -0.0384615, 0.0102564, 0.0589744, 0.107692, 0.15641, 0.205128, 0.253846, 0.302564, 0.351282, 0.4]
  out "Current Device":u32=10
  out "Total Device":u32=10
  out "IV fine log":cluster{dbl[], dbl[]}[](graph)=[{[-1.5, -1.45128, -1.40256, -1.35385, -1.30513, -1.25641, -1.20769, -1.15897, -1.11026, -1.06154, -1.01282, -0.964103, -0.915385, -0.866667, -0.817949, -0.769231, -0.720513, -0.671795, -0.623077, -0.574359, -0.525641, -0.476923, -0.428205, -0.379487, -0.330769, -0.282051, -0.233333, -0.184615, -0.135897, -0.0871795, -0.0384615, 0.0102564, 0.0589744, 0.107692, 0.15641, 0.205128, 0.253846, 0.302564, 0.351282, 0.4], [1.62518e-05, 1.59058e-05, 1.58552e-05, 1.58521e-05, 1.61136e-05, 1.58325e-05, 1.57837e-05, 1.57923e-05, 1.59421e-05, 1.57195e-05, 1.57072e-05, 1.57655e-05, 1.57462e-05, 1.56593e-05, 1.55775e-05, 1.56026e-05, 1.55346e-05, 1.54639e-05, 1.53912e-05, 1.53075e-05, 1.51382e-05, 1.50399e-05, 1.4928e-05, 1.47321e-05, 1.44447e-05, 1.42751e-05, 1.40992e-05, 1.37417e-05, 1.3347e-05, 1.30217e-05, 1.26796e-05, 1.21766e-05, 1.16136e-05, 1.09335e-05, 1.00961e-05, 8.60584e-06, 7.26446e-06, 4.26576e-06, 1.99124e-06, 1.66138e-05]}, {[-1.5, -1.45128, -1.40256, -1.35385, -1.30513, -1.25641, -1.20769, -1.15897, -1.11026, -1.06154, -1.01282, -0.964103, -0.915385, -0.866667, -0.817949, -0.769231, -0.720513, -0.671795, -0.623077, -0.574359, -0.525641, -0.476923, -0.428205, -0.379487, -0.330769, -0.282051, -0.233333, -0.184615, -0.135897, -0.0871795, -0.0384615, 0.0102564, 0.0589744, 0.107692, 0.15641, 0.205128, 0.253846, 0.302564, 0.351282, 0.4], [1.36029e-05, 1.39238e-05, 1.40077e-05, 1.39787e-05, 1.37902e-05, 1.38254e-05, 1.38807e-05, 1.39993e-05, 1.37559e-05, 1.37594e-05, 1.39334e-05, 1.38859e-05, 1.37374e-05, 1.37784e-05, 1.38315e-05, 1.3849e-05, 1.36736e-05, 1.36255e-05, 1.36181e-05, 1.35913e-05, 1.34346e-05, 1.33435e-05, 1.31651e-05, 1.30411e-05, 1.28623e-05, 1.27277e-05, 1.24139e-05, 1.2144e-05, 1.18426e-05, 1.15662e-05, 1.11112e-05, 1.06968e-05, 1.02089e-05, 9.22437e-06, 8.85657e-06, 7.82706e-06, 6.25243e-06, 3.38221e-06, 2.74369e-06, 1.77865e-05]}, {[-1.5, -1.45128, -1.40256, -1.35385, -1.30513, -1.25641, -1.20769, -1.15897, -1.11026, -1.06154, -1.01282, -0.964103, -0.915385, -0.866667, -0.817949, -0.769231, -0.720513, -0.671795, -0.623077, -0.574359, -0.525641, -0.476923, -0.428205, -0.379487, -0.330769, -0.282051, -0.233333, -0.184615, -0.135897, -0.0871795, -0.0384615, 0.0102564, 0.0589744, 0.107692, 0.15641, 0.205128, 0.253846, 0.302564, 0.351282, 0.4], [1.45487e-05, 1.44793e-05, 1.45091e-05, 1.45759e-05, 1.44845e-05, 1.44589e-05, 1.44101e-05, 1.43467e-05, 1.42634e-05, 1.42416e-05, 1.41538e-05, 1.39764e-05, 1.38688e-05, 1.37779e-05, 1.3677e-05, 1.34647e-05, 1.3336e-05, 1.32085e-05, 1.30882e-05, 1.28545e-05, 1.26536e-05, 1.24643e-05, 1.22342e-05, 1.20329e-05, 1.17647e-05, 1.14825e-05, 1.12311e-05, 1.09497e-05, 1.06108e-05, 1.02268e-05, 9.51786e-06, 9.44586e-06, 8.95039e-06, 8.37403e-06, 7.69201e-06, 6.79217e-06, 5.3745e-06, 2.81715e-06, 2.94395e-06, 1.74863e-05]}, {[-1.5, -1.45128, -1.40256, -1.35385, -1.30513, -1.25641, -1.20769, -1.15897, -1.11026, -1.06154, -1.01282, -0.964103, -0.915385, -0.866667, -0.817949, -0.769231, -0.720513, -0.671795, -0.623077, -0.574359, -0.525641, -0.476923, -0.428205, -0.379487, -0.330769, -0.282051, -0.233333, -0.184615, -0.135897, -0.0871795, -0.0384615, 0.0102564, 0.0589744, 0.107692, 0.15641, 0.205128, 0.253846, 0.302564, 0.351282, 0.4], [1.43268e-05, 1.41291e-05, 1.40792e-05, 1.40388e-05, 1.41617e-05, 1.40803e-05, 1.40236e-05, 1.39445e-05, 1.39384e-05, 1.3893e-05, 1.38786e-05, 1.38031e-05, 1.37261e-05, 1.37001e-05, 1.35949e-05, 1.3466e-05, 1.33568e-05, 1.31818e-05, 1.30797e-05, 1.28908e-05, 1.2725e-05, 1.25568e-05, 1.23307e-05, 1.21443e-05, 1.19645e-05, 1.17361e-05, 1.14207e-05, 1.11251e-05, 1.08126e-05, 1.04759e-05, 1.01039e-05, 9.29569e-06, 9.16141e-06, 8.54072e-06, 7.80004e-06, 6.80414e-06, 5.32019e-06, 2.59009e-06, 3.20517e-06, 1.73178e-05]}, {[-1.5, -1.45128, -1.40256, -1.35385, -1.30513, -1.25641, -1.20769, -1.15897, -1.11026, -1.06154, -1.01282, -0.964103, -0.915385, -0.866667, -0.817949, -0.769231, -0.720513, -0.671795, -0.623077, -0.574359, -0.525641, -0.476923, -0.428205, -0.379487, -0.330769, -0.282051, -0.233333, -0.184615, -0.135897, -0.0871795, -0.0384615, 0.0102564, 0.0589744, 0.107692, 0.15641, 0.205128, 0.253846, 0.302564, 0.351282, 0.4], [1.45128e-05, 1.44784e-05, 1.44337e-05, 1.45008e-05, 1.44765e-05, 1.44197e-05, 1.44825e-05, 1.44147e-05, 1.44257e-05, 1.44417e-05, 1.44472e-05, 1.43745e-05, 1.43881e-05, 1.43696e-05, 1.43656e-05, 1.44001e-05, 1.4292e-05, 1.43096e-05, 1.42966e-05, 1.42992e-05, 1.42272e-05, 1.41855e-05, 1.40808e-05, 1.39327e-05, 1.38064e-05, 1.37047e-05, 1.34936e-05, 1.32621e-05, 1.30014e-05, 1.26801e-05, 1.23085e-05, 1.18747e-05, 1.12903e-05, 1.06544e-05, 9.40974e-06, 8.59154e-06, 6.76655e-06, 3.48424e-06, 3.40767e-06, 1.98841e-05]}, {[-1.5, -1.45128, -1.40256, -1.35385, -1.30513, -1.25641, -1.20769, -1.15897, -1.11026, -1.06154, -1.01282, -0.964103, -0.915385, -0.866667, -0.817949, -0.769231, -0.720513, -0.671795, -0.623077, -0.574359, -0.525641, -0.476923, -0.428205, -0.379487, -0.330769, -0.282051, -0.233333, -0.184615, -0.135897, -0.0871795, -0.0384615, 0.0102564, 0.0589744, 0.107692, 0.15641, 0.205128, 0.253846, 0.302564, 0.351282, 0.4], [1.40475e-05, 1.4354e-05, 1.44564e-05, 1.44012e-05, 1.42809e-05, 1.43571e-05, 1.43786e-05, 1.43287e-05, 1.42537e-05, 1.42975e-05, 1.43208e-05, 1.42332e-05, 1.41469e-05, 1.41822e-05, 1.42689e-05, 1.42063e-05, 1.40896e-05, 1.39596e-05, 1.39855e-05, 1.39085e-05, 1.37852e-05, 1.36034e-05, 1.34773e-05, 1.33117e-05, 1.30942e-05, 1.28233e-05, 1.25734e-05, 1.22817e-05, 1.19194e-05, 1.16165e-05, 1.11835e-05, 1.07278e-05, 1.02202e-05, 9.20555e-06, 8.77193e-06, 7.70772e-06, 6.0801e-06, 3.16101e-06, 3.17945e-06, 1.88686e-05]}, {[-1.5, -1.45128, -1.40256, -1.35385, -1.30513, -1.25641, -1.20769, -1.15897, -1.11026, -1.06154, -1.01282, -0.964103, -0.915385, -0.866667, -0.817949, -0.769231, -0.720513, -0.671795, -0.623077, -0.574359, -0.525641, -0.476923, -0.428205, -0.379487, -0.330769, -0.282051, -0.233333, -0.184615, -0.135897, -0.0871795, -0.0384615, 0.0102564, 0.0589744, 0.107692, 0.15641, 0.205128, 0.253846, 0.302564, 0.351282, 0.4], [1.54351e-05, 1.50601e-05, 1.51056e-05, 1.52663e-05, 1.52168e-05, 1.51171e-05, 1.507e-05, 1.51743e-05, 1.51078e-05, 1.50298e-05, 1.49971e-05, 1.49526e-05, 1.49294e-05, 1.48765e-05, 1.46879e-05, 1.45901e-05, 1.44709e-05, 1.43723e-05, 1.41737e-05, 1.39806e-05, 1.37765e-05, 1.36025e-05, 1.338e-05, 1.30992e-05, 1.28407e-05, 1.25943e-05, 1.22959e-05, 1.19637e-05, 1.16023e-05, 1.12135e-05, 1.08209e-05, 1.03236e-05, 9.4587e-06, 9.22359e-06, 8.4509e-06, 7.48066e-06, 5.98309e-06, 3.29111e-06, 2.65596e-06, 1.74357e-05]}, {[-1.5, -1.45128, -1.40256, -1.35385, -1.30513, -1.25641, -1.20769, -1.15897, -1.11026, -1.06154, -1.01282, -0.964103, -0.915385, -0.866667, -0.817949, -0.769231, -0.720513, -0.671795, -0.623077, -0.574359, -0.525641, -0.476923, -0.428205, -0.379487, -0.330769, -0.282051, -0.233333, -0.184615, -0.135897, -0.0871795, -0.0384615, 0.0102564, 0.0589744, 0.107692, 0.15641, 0.205128, 0.253846, 0.302564, 0.351282, 0.4], [1.53447e-05, 1.47831e-05, 1.47122e-05, 1.46429e-05, 1.47243e-05, 1.47328e-05, 1.47086e-05, 1.46028e-05, 1.47432e-05, 1.47113e-05, 1.47218e-05, 1.46376e-05, 1.46699e-05, 1.46152e-05, 1.46717e-05, 1.46125e-05, 1.45853e-05, 1.46234e-05, 1.45533e-05, 1.44673e-05, 1.44896e-05, 1.4478e-05, 1.4459e-05, 1.43998e-05, 1.43584e-05, 1.425e-05, 1.42328e-05, 1.40931e-05, 1.38244e-05, 1.35004e-05, 1.31121e-05, 1.26449e-05, 1.20102e-05, 1.12588e-05, 1.02839e-05, 8.58833e-06, 6.90248e-06, 3.40666e-06, 3.80601e-06, 2.08878e-05]}, {[-1.5, -1.45128, -1.40256, -1.35385, -1.30513, -1.25641, -1.20769, -1.15897, -1.11026, -1.06154, -1.01282, -0.964103, -0.915385, -0.866667, -0.817949, -0.769231, -0.720513, -0.671795, -0.623077, -0.574359, -0.525641, -0.476923, -0.428205, -0.379487, -0.330769, -0.282051, -0.233333, -0.184615, -0.135897, -0.0871795, -0.0384615, 0.0102564, 0.0589744, 0.107692, 0.15641, 0.205128, 0.253846, 0.302564, 0.351282, 0.4], [1.44727e-05, 1.4384e-05, 1.44688e-05, 1.43704e-05, 1.43565e-05, 1.44014e-05, 1.44225e-05, 1.44796e-05, 1.43648e-05, 1.4355e-05, 1.43902e-05, 1.4375e-05, 1.43596e-05, 1.42258e-05, 1.43194e-05, 1.43306e-05, 1.42962e-05, 1.41932e-05, 1.41703e-05, 1.40789e-05, 1.41097e-05, 1.39534e-05, 1.39183e-05, 1.38152e-05, 1.36883e-05, 1.34469e-05, 1.32306e-05, 1.29288e-05, 1.27267e-05, 1.23973e-05, 1.19846e-05, 1.14551e-05, 1.08658e-05, 1.01658e-05, 8.93522e-06, 8.01026e-06, 6.20114e-06, 2.94987e-06, 3.83666e-06, 2.00962e-05]}, {[-1.5, -1.45128, -1.40256, -1.35385, -1.30513, -1.25641, -1.20769, -1.15897, -1.11026, -1.06154, -1.01282, -0.964103, -0.915385, -0.866667, -0.817949, -0.769231, -0.720513, -0.671795, -0.623077, -0.574359, -0.525641, -0.476923, -0.428205, -0.379487, -0.330769, -0.282051, -0.233333, -0.184615, -0.135897, -0.0871795, -0.0384615, 0.0102564, 0.0589744, 0.107692, 0.15641, 0.205128, 0.253846, 0.302564, 0.351282, 0.4], [1.52182e-05, 1.47166e-05, 1.48638e-05, 1.4948e-05, 1.49634e-05, 1.49403e-05, 1.48575e-05, 1.48749e-05, 1.47754e-05, 1.47251e-05, 1.46559e-05, 1.45851e-05, 1.45028e-05, 1.43852e-05, 1.42468e-05, 1.41684e-05, 1.40308e-05, 1.39364e-05, 1.37397e-05, 1.35679e-05, 1.3482e-05, 1.32093e-05, 1.2996e-05, 1.28281e-05, 1.25632e-05, 1.23417e-05, 1.20643e-05, 1.17371e-05, 1.14516e-05, 1.10657e-05, 1.06617e-05, 1.02025e-05, 9.26216e-06, 9.00798e-06, 8.21814e-06, 7.12779e-06, 5.50195e-06, 2.50105e-06, 4.02524e-06, 2.01571e-05]}]
  out "Progress 2":u8(slide)=100 scale=0.0..100.0
  in  "StartFine":bool
  out "IV fine linear":cluster{dbl[], dbl[]}[](graph)=[{[-1.5, -1.45128, -1.40256, -1.35385, -1.30513, -1.25641, -1.20769, -1.15897, -1.11026, -1.06154, -1.01282, -0.964103, -0.915385, -0.866667, -0.817949, -0.769231, -0.720513, -0.671795, -0.623077, -0.574359, -0.525641, -0.476923, -0.428205, -0.379487, -0.330769, -0.282051, -0.233333, -0.184615, -0.135897, -0.0871795, -0.0384615, 0.0102564, 0.0589744, 0.107692, 0.15641, 0.205128, 0.253846, 0.302564, 0.351282, 0.4], [-1.62518e-05, -1.59058e-05, -1.58552e-05, -1.58521e-05, -1.61136e-05, -1.58325e-05, -1.57837e-05, -1.57923e-05, -1.59421e-05, -1.57195e-05, -1.57072e-05, -1.57655e-05, -1.57462e-05, -1.56593e-05, -1.55775e-05, -1.56026e-05, -1.55346e-05, -1.54639e-05, -1.53912e-05, -1.53075e-05, -1.51382e-05, -1.50399e-05, -1.4928e-05, -1.47321e-05, -1.44447e-05, -1.42751e-05, -1.40992e-05, -1.37417e-05, -1.3347e-05, -1.30217e-05, -1.26796e-05, -1.21766e-05, -1.16136e-05, -1.09335e-05, -1.00961e-05, -8.60584e-06, -7.26446e-06, -4.26576e-06, 1.99124e-06, 1.66138e-05]}, {[-1.5, -1.45128, -1.40256, -1.35385, -1.30513, -1.25641, -1.20769, -1.15897, -1.11026, -1.06154, -1.01282, -0.964103, -0.915385, -0.866667, -0.817949, -0.769231, -0.720513, -0.671795, -0.623077, -0.574359, -0.525641, -0.476923, -0.428205, -0.379487, -0.330769, -0.282051, -0.233333, -0.184615, -0.135897, -0.0871795, -0.0384615, 0.0102564, 0.0589744, 0.107692, 0.15641, 0.205128, 0.253846, 0.302564, 0.351282, 0.4], [-1.36029e-05, -1.39238e-05, -1.40077e-05, -1.39787e-05, -1.37902e-05, -1.38254e-05, -1.38807e-05, -1.39993e-05, -1.37559e-05, -1.37594e-05, -1.39334e-05, -1.38859e-05, -1.37374e-05, -1.37784e-05, -1.38315e-05, -1.3849e-05, -1.36736e-05, -1.36255e-05, -1.36181e-05, -1.35913e-05, -1.34346e-05, -1.33435e-05, -1.31651e-05, -1.30411e-05, -1.28623e-05, -1.27277e-05, -1.24139e-05, -1.2144e-05, -1.18426e-05, -1.15662e-05, -1.11112e-05, -1.06968e-05, -1.02089e-05, -9.22437e-06, -8.85657e-06, -7.82706e-06, -6.25243e-06, -3.38221e-06, 2.74369e-06, 1.77865e-05]}, {[-1.5, -1.45128, -1.40256, -1.35385, -1.30513, -1.25641, -1.20769, -1.15897, -1.11026, -1.06154, -1.01282, -0.964103, -0.915385, -0.866667, -0.817949, -0.769231, -0.720513, -0.671795, -0.623077, -0.574359, -0.525641, -0.476923, -0.428205, -0.379487, -0.330769, -0.282051, -0.233333, -0.184615, -0.135897, -0.0871795, -0.0384615, 0.0102564, 0.0589744, 0.107692, 0.15641, 0.205128, 0.253846, 0.302564, 0.351282, 0.4], [-1.45487e-05, -1.44793e-05, -1.45091e-05, -1.45759e-05, -1.44845e-05, -1.44589e-05, -1.44101e-05, -1.43467e-05, -1.42634e-05, -1.42416e-05, -1.41538e-05, -1.39764e-05, -1.38688e-05, -1.37779e-05, -1.3677e-05, -1.34647e-05, -1.3336e-05, -1.32085e-05, -1.30882e-05, -1.28545e-05, -1.26536e-05, -1.24643e-05, -1.22342e-05, -1.20329e-05, -1.17647e-05, -1.14825e-05, -1.12311e-05, -1.09497e-05, -1.06108e-05, -1.02268e-05, -9.51786e-06, -9.44586e-06, -8.95039e-06, -8.37403e-06, -7.69201e-06, -6.79217e-06, -5.3745e-06, -2.81715e-06, 2.94395e-06, 1.74863e-05]}, {[-1.5, -1.45128, -1.40256, -1.35385, -1.30513, -1.25641, -1.20769, -1.15897, -1.11026, -1.06154, -1.01282, -0.964103, -0.915385, -0.866667, -0.817949, -0.769231, -0.720513, -0.671795, -0.623077, -0.574359, -0.525641, -0.476923, -0.428205, -0.379487, -0.330769, -0.282051, -0.233333, -0.184615, -0.135897, -0.0871795, -0.0384615, 0.0102564, 0.0589744, 0.107692, 0.15641, 0.205128, 0.253846, 0.302564, 0.351282, 0.4], [-1.43268e-05, -1.41291e-05, -1.40792e-05, -1.40388e-05, -1.41617e-05, -1.40803e-05, -1.40236e-05, -1.39445e-05, -1.39384e-05, -1.3893e-05, -1.38786e-05, -1.38031e-05, -1.37261e-05, -1.37001e-05, -1.35949e-05, -1.3466e-05, -1.33568e-05, -1.31818e-05, -1.30797e-05, -1.28908e-05, -1.2725e-05, -1.25568e-05, -1.23307e-05, -1.21443e-05, -1.19645e-05, -1.17361e-05, -1.14207e-05, -1.11251e-05, -1.08126e-05, -1.04759e-05, -1.01039e-05, -9.29569e-06, -9.16141e-06, -8.54072e-06, -7.80004e-06, -6.80414e-06, -5.32019e-06, -2.59009e-06, 3.20517e-06, 1.73178e-05]}, {[-1.5, -1.45128, -1.40256, -1.35385, -1.30513, -1.25641, -1.20769, -1.15897, -1.11026, -1.06154, -1.01282, -0.964103, -0.915385, -0.866667, -0.817949, -0.769231, -0.720513, -0.671795, -0.623077, -0.574359, -0.525641, -0.476923, -0.428205, -0.379487, -0.330769, -0.282051, -0.233333, -0.184615, -0.135897, -0.0871795, -0.0384615, 0.0102564, 0.0589744, 0.107692, 0.15641, 0.205128, 0.253846, 0.302564, 0.351282, 0.4], [-1.45128e-05, -1.44784e-05, -1.44337e-05, -1.45008e-05, -1.44765e-05, -1.44197e-05, -1.44825e-05, -1.44147e-05, -1.44257e-05, -1.44417e-05, -1.44472e-05, -1.43745e-05, -1.43881e-05, -1.43696e-05, -1.43656e-05, -1.44001e-05, -1.4292e-05, -1.43096e-05, -1.42966e-05, -1.42992e-05, -1.42272e-05, -1.41855e-05, -1.40808e-05, -1.39327e-05, -1.38064e-05, -1.37047e-05, -1.34936e-05, -1.32621e-05, -1.30014e-05, -1.26801e-05, -1.23085e-05, -1.18747e-05, -1.12903e-05, -1.06544e-05, -9.40974e-06, -8.59154e-06, -6.76655e-06, -3.48424e-06, 3.40767e-06, 1.98841e-05]}, {[-1.5, -1.45128, -1.40256, -1.35385, -1.30513, -1.25641, -1.20769, -1.15897, -1.11026, -1.06154, -1.01282, -0.964103, -0.915385, -0.866667, -0.817949, -0.769231, -0.720513, -0.671795, -0.623077, -0.574359, -0.525641, -0.476923, -0.428205, -0.379487, -0.330769, -0.282051, -0.233333, -0.184615, -0.135897, -0.0871795, -0.0384615, 0.0102564, 0.0589744, 0.107692, 0.15641, 0.205128, 0.253846, 0.302564, 0.351282, 0.4], [-1.40475e-05, -1.4354e-05, -1.44564e-05, -1.44012e-05, -1.42809e-05, -1.43571e-05, -1.43786e-05, -1.43287e-05, -1.42537e-05, -1.42975e-05, -1.43208e-05, -1.42332e-05, -1.41469e-05, -1.41822e-05, -1.42689e-05, -1.42063e-05, -1.40896e-05, -1.39596e-05, -1.39855e-05, -1.39085e-05, -1.37852e-05, -1.36034e-05, -1.34773e-05, -1.33117e-05, -1.30942e-05, -1.28233e-05, -1.25734e-05, -1.22817e-05, -1.19194e-05, -1.16165e-05, -1.11835e-05, -1.07278e-05, -1.02202e-05, -9.20555e-06, -8.77193e-06, -7.70772e-06, -6.0801e-06, -3.16101e-06, 3.17945e-06, 1.88686e-05]}, {[-1.5, -1.45128, -1.40256, -1.35385, -1.30513, -1.25641, -1.20769, -1.15897, -1.11026, -1.06154, -1.01282, -0.964103, -0.915385, -0.866667, -0.817949, -0.769231, -0.720513, -0.671795, -0.623077, -0.574359, -0.525641, -0.476923, -0.428205, -0.379487, -0.330769, -0.282051, -0.233333, -0.184615, -0.135897, -0.0871795, -0.0384615, 0.0102564, 0.0589744, 0.107692, 0.15641, 0.205128, 0.253846, 0.302564, 0.351282, 0.4], [-1.54351e-05, -1.50601e-05, -1.51056e-05, -1.52663e-05, -1.52168e-05, -1.51171e-05, -1.507e-05, -1.51743e-05, -1.51078e-05, -1.50298e-05, -1.49971e-05, -1.49526e-05, -1.49294e-05, -1.48765e-05, -1.46879e-05, -1.45901e-05, -1.44709e-05, -1.43723e-05, -1.41737e-05, -1.39806e-05, -1.37765e-05, -1.36025e-05, -1.338e-05, -1.30992e-05, -1.28407e-05, -1.25943e-05, -1.22959e-05, -1.19637e-05, -1.16023e-05, -1.12135e-05, -1.08209e-05, -1.03236e-05, -9.4587e-06, -9.22359e-06, -8.4509e-06, -7.48066e-06, -5.98309e-06, -3.29111e-06, 2.65596e-06, 1.74357e-05]}, {[-1.5, -1.45128, -1.40256, -1.35385, -1.30513, -1.25641, -1.20769, -1.15897, -1.11026, -1.06154, -1.01282, -0.964103, -0.915385, -0.866667, -0.817949, -0.769231, -0.720513, -0.671795, -0.623077, -0.574359, -0.525641, -0.476923, -0.428205, -0.379487, -0.330769, -0.282051, -0.233333, -0.184615, -0.135897, -0.0871795, -0.0384615, 0.0102564, 0.0589744, 0.107692, 0.15641, 0.205128, 0.253846, 0.302564, 0.351282, 0.4], [-1.53447e-05, -1.47831e-05, -1.47122e-05, -1.46429e-05, -1.47243e-05, -1.47328e-05, -1.47086e-05, -1.46028e-05, -1.47432e-05, -1.47113e-05, -1.47218e-05, -1.46376e-05, -1.46699e-05, -1.46152e-05, -1.46717e-05, -1.46125e-05, -1.45853e-05, -1.46234e-05, -1.45533e-05, -1.44673e-05, -1.44896e-05, -1.4478e-05, -1.4459e-05, -1.43998e-05, -1.43584e-05, -1.425e-05, -1.42328e-05, -1.40931e-05, -1.38244e-05, -1.35004e-05, -1.31121e-05, -1.26449e-05, -1.20102e-05, -1.12588e-05, -1.02839e-05, -8.58833e-06, -6.90248e-06, -3.40666e-06, 3.80601e-06, 2.08878e-05]}, {[-1.5, -1.45128, -1.40256, -1.35385, -1.30513, -1.25641, -1.20769, -1.15897, -1.11026, -1.06154, -1.01282, -0.964103, -0.915385, -0.866667, -0.817949, -0.769231, -0.720513, -0.671795, -0.623077, -0.574359, -0.525641, -0.476923, -0.428205, -0.379487, -0.330769, -0.282051, -0.233333, -0.184615, -0.135897, -0.0871795, -0.0384615, 0.0102564, 0.0589744, 0.107692, 0.15641, 0.205128, 0.253846, 0.302564, 0.351282, 0.4], [-1.44727e-05, -1.4384e-05, -1.44688e-05, -1.43704e-05, -1.43565e-05, -1.44014e-05, -1.44225e-05, -1.44796e-05, -1.43648e-05, -1.4355e-05, -1.43902e-05, -1.4375e-05, -1.43596e-05, -1.42258e-05, -1.43194e-05, -1.43306e-05, -1.42962e-05, -1.41932e-05, -1.41703e-05, -1.40789e-05, -1.41097e-05, -1.39534e-05, -1.39183e-05, -1.38152e-05, -1.36883e-05, -1.34469e-05, -1.32306e-05, -1.29288e-05, -1.27267e-05, -1.23973e-05, -1.19846e-05, -1.14551e-05, -1.08658e-05, -1.01658e-05, -8.93522e-06, -8.01026e-06, -6.20114e-06, -2.94987e-06, 3.83666e-06, 2.00962e-05]}, {[-1.5, -1.45128, -1.40256, -1.35385, -1.30513, -1.25641, -1.20769, -1.15897, -1.11026, -1.06154, -1.01282, -0.964103, -0.915385, -0.866667, -0.817949, -0.769231, -0.720513, -0.671795, -0.623077, -0.574359, -0.525641, -0.476923, -0.428205, -0.379487, -0.330769, -0.282051, -0.233333, -0.184615, -0.135897, -0.0871795, -0.0384615, 0.0102564, 0.0589744, 0.107692, 0.15641, 0.205128, 0.253846, 0.302564, 0.351282, 0.4], [-1.52182e-05, -1.47166e-05, -1.48638e-05, -1.4948e-05, -1.49634e-05, -1.49403e-05, -1.48575e-05, -1.48749e-05, -1.47754e-05, -1.47251e-05, -1.46559e-05, -1.45851e-05, -1.45028e-05, -1.43852e-05, -1.42468e-05, -1.41684e-05, -1.40308e-05, -1.39364e-05, -1.37397e-05, -1.35679e-05, -1.3482e-05, -1.32093e-05, -1.2996e-05, -1.28281e-05, -1.25632e-05, -1.23417e-05, -1.20643e-05, -1.17371e-05, -1.14516e-05, -1.10657e-05, -1.06617e-05, -1.02025e-05, -9.26216e-06, -9.00798e-06, -8.21814e-06, -7.12779e-06, -5.50195e-06, -2.50105e-06, 4.02524e-06, 2.01571e-05]}]
  in  "Mask File Fine":path=path "C:/Users/Flash/Desktop/Data/Detector test data/SL066_mask_map_file_V3_align on D3000_Diode_Open_1000_A-3348-2-A_1000123103_040000.0PM.csv"
  in  "Prober GPIB":string="0:1"
  in  "SMU":refnum<visa-resource-name>="GPIB0::26::INSTR"
  in  "Channel":enum32{"Channel A", "Channel B"}(ring)
  # "0 is for dark IV!"
  # "Sweep Settings"
  # "Forward Voltage"
  # "Dark/Light Current"
  # "Check settings before click start!"
  # "Make sure current x and y are same as prober before click Start!"
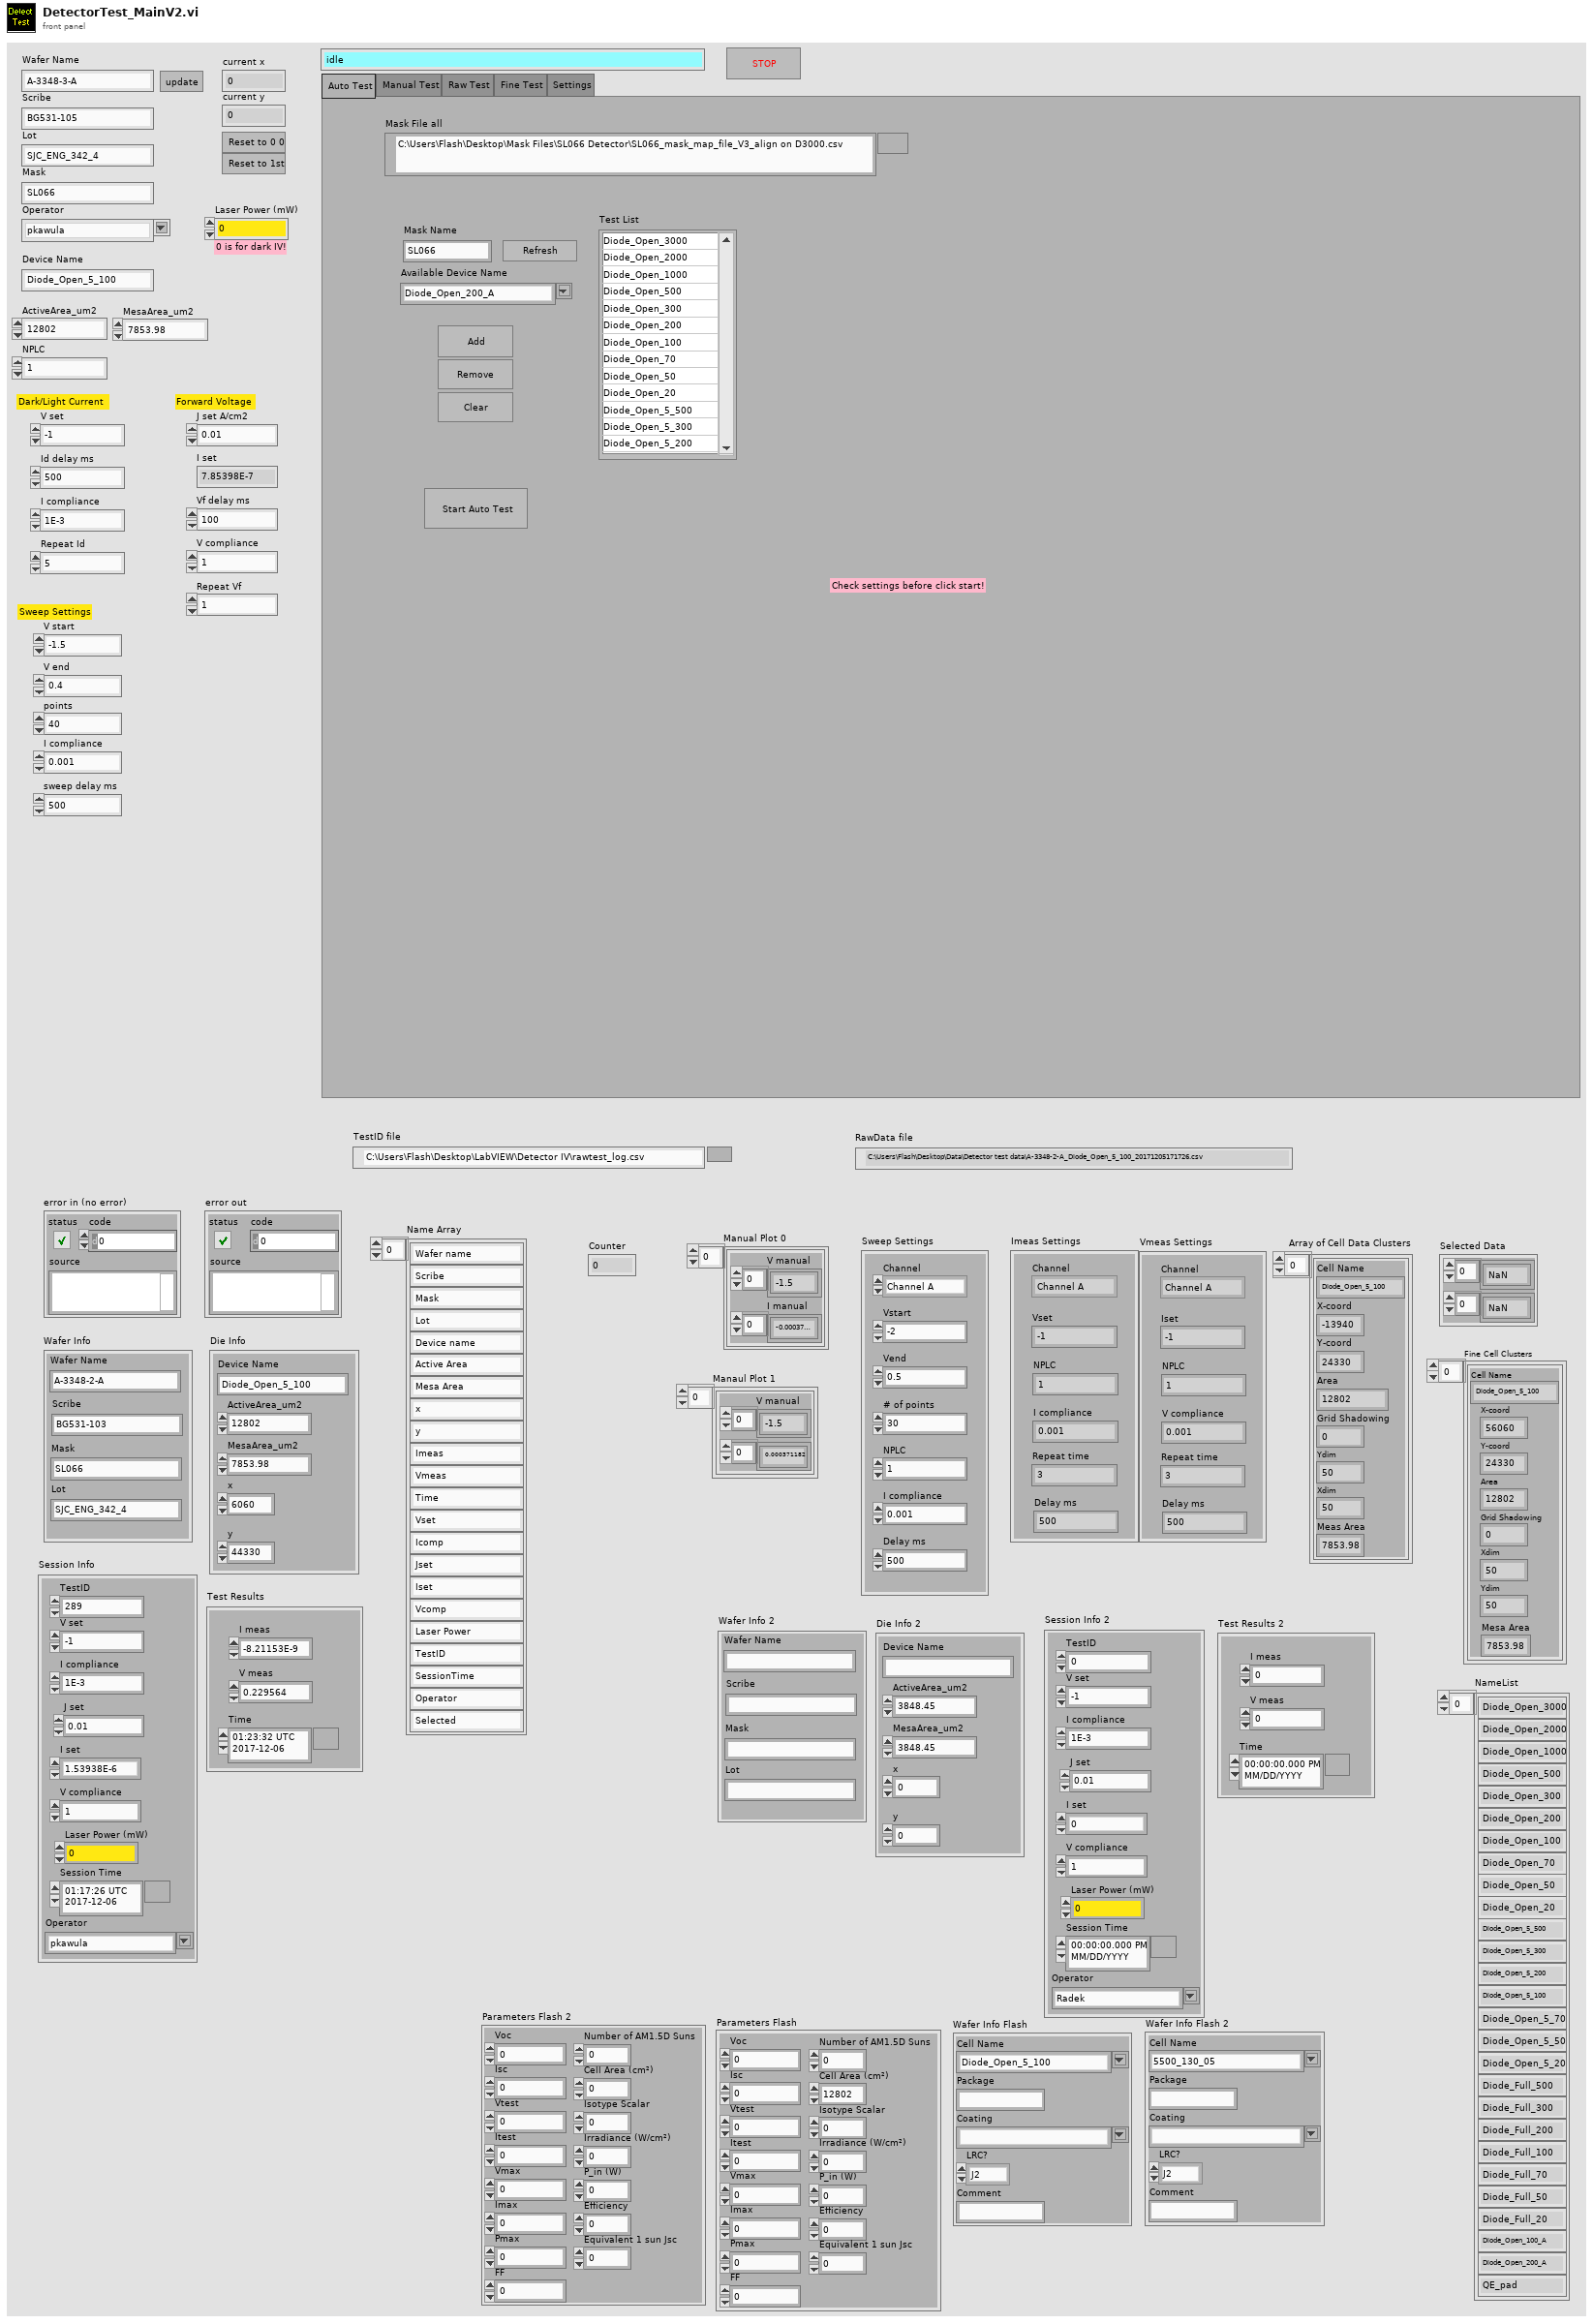
[diagram p1: front panel]
types:
  T1 = cluster{"Cell Name":string, "Package":string, "Coating":string, "LRC?":enum16{"J1", "J2", "LRC"}, "Comment":string}
  T2 = cluster{"Voc":dbl, "Isc":dbl, "FF":dbl, "Vtest":dbl, "Imax":dbl, "Vmax":dbl, "Pmax":dbl, "Itest":dbl, "Efficiency":dbl, "P_in (W)":dbl, "Irradiance (W/cm²)":dbl, "Cell Area (cm²)":dbl, "Number of AM1.5D Suns":dbl, "Isotype Scalar":dbl, "Equivalent 1 sun Jsc":dbl}
  T3 = cluster{"Cell Name":string, "X-coord":dbl, "Y-coord":dbl, "Area":dbl, "Grid Shadowing":dbl, "Xdim":dbl, "Ydim":dbl, "Mesa Area":dbl}[]
  T4 = cluster{"I meas":dbl, "V meas":dbl, "Time":timestamp}
  T5 = cluster{"V set":dbl, "I compliance":dbl, "J set":dbl, "I set":dbl, "V compliance":dbl, "Laser Power (mW)":dbl, "TestID":u32, "Session Time":timestamp, "Operator":string}
  T6 = cluster{"Device Name":string, "ActiveArea_um2":dbl, "MesaArea_um2":dbl, "x":dbl, "y":dbl}
  T7 = cluster{"Wafer Name":string, "Scribe":string, "Mask":string, "Lot":string}
  T8 = cluster{"Channel":enum32{"Channel A", "Channel B"}, "Vstart":dbl, "Vend":dbl, "# of points":u16, "NPLC":dbl, "I compliance":dbl, "Delay ms":dbl}
  T9 = cluster{"Channel":enum32{"Channel A", "Channel B"}, "Iset":dbl, "NPLC":dbl, "V compliance":dbl, "Repeat time":u16, "Delay ms":dbl}
  T10 = cluster{"Channel":enum32{"Channel A", "Channel B"}, "Vset":dbl, "NPLC":dbl, "I compliance":dbl, "Repeat time":u16, "Delay ms":dbl}
  T11 = cluster{"Cell Name":string, "X-coord":dbl, "Y-coord":dbl, "Area":dbl, "Grid Shadowing":dbl, "Ydim":dbl, "Xdim":dbl, "Meas Area":dbl}[]
  T12 = enum32{"Auto Test", "Manual Test", "Raw Test", "Fine Test", "Settings"}
  T13 = cluster{"X Values":dbl[], "Histogram: h(x)":i32[]}
  T14 = cluster{"Cell Name":string, "X-coord":dbl, "Y-coord":dbl, "Area":dbl, "Grid Shadowing":dbl, "Ydim":dbl, "Xdim":dbl, "Meas Area":dbl}
  T15 = cluster{"Varray manual":dbl[], "Iarray manual":dbl[]}[]
  T16 = cluster{"WaferName":string, "Scribe":string, "Structure":string, "Lot":string, "Mask":string}
  T17 = cluster{"V set":dbl, "I compliance":dbl, "J set":dbl, "I set":dbl, "V compliance":dbl, "Laser Power (mW)":dbl, "TestID":u32, "Operator":string}
  T18 = cluster{"Device Name":string, "ActiveArea_um2":dbl, "MesaArea_um2":dbl}
  T19 = cluster{"Cell Name":string, "X-coord":dbl, "Y-coord":dbl, "Area":dbl, "Grid Shadowing":dbl, "Xdim":dbl, "Ydim":dbl, "Mesa Area":dbl}
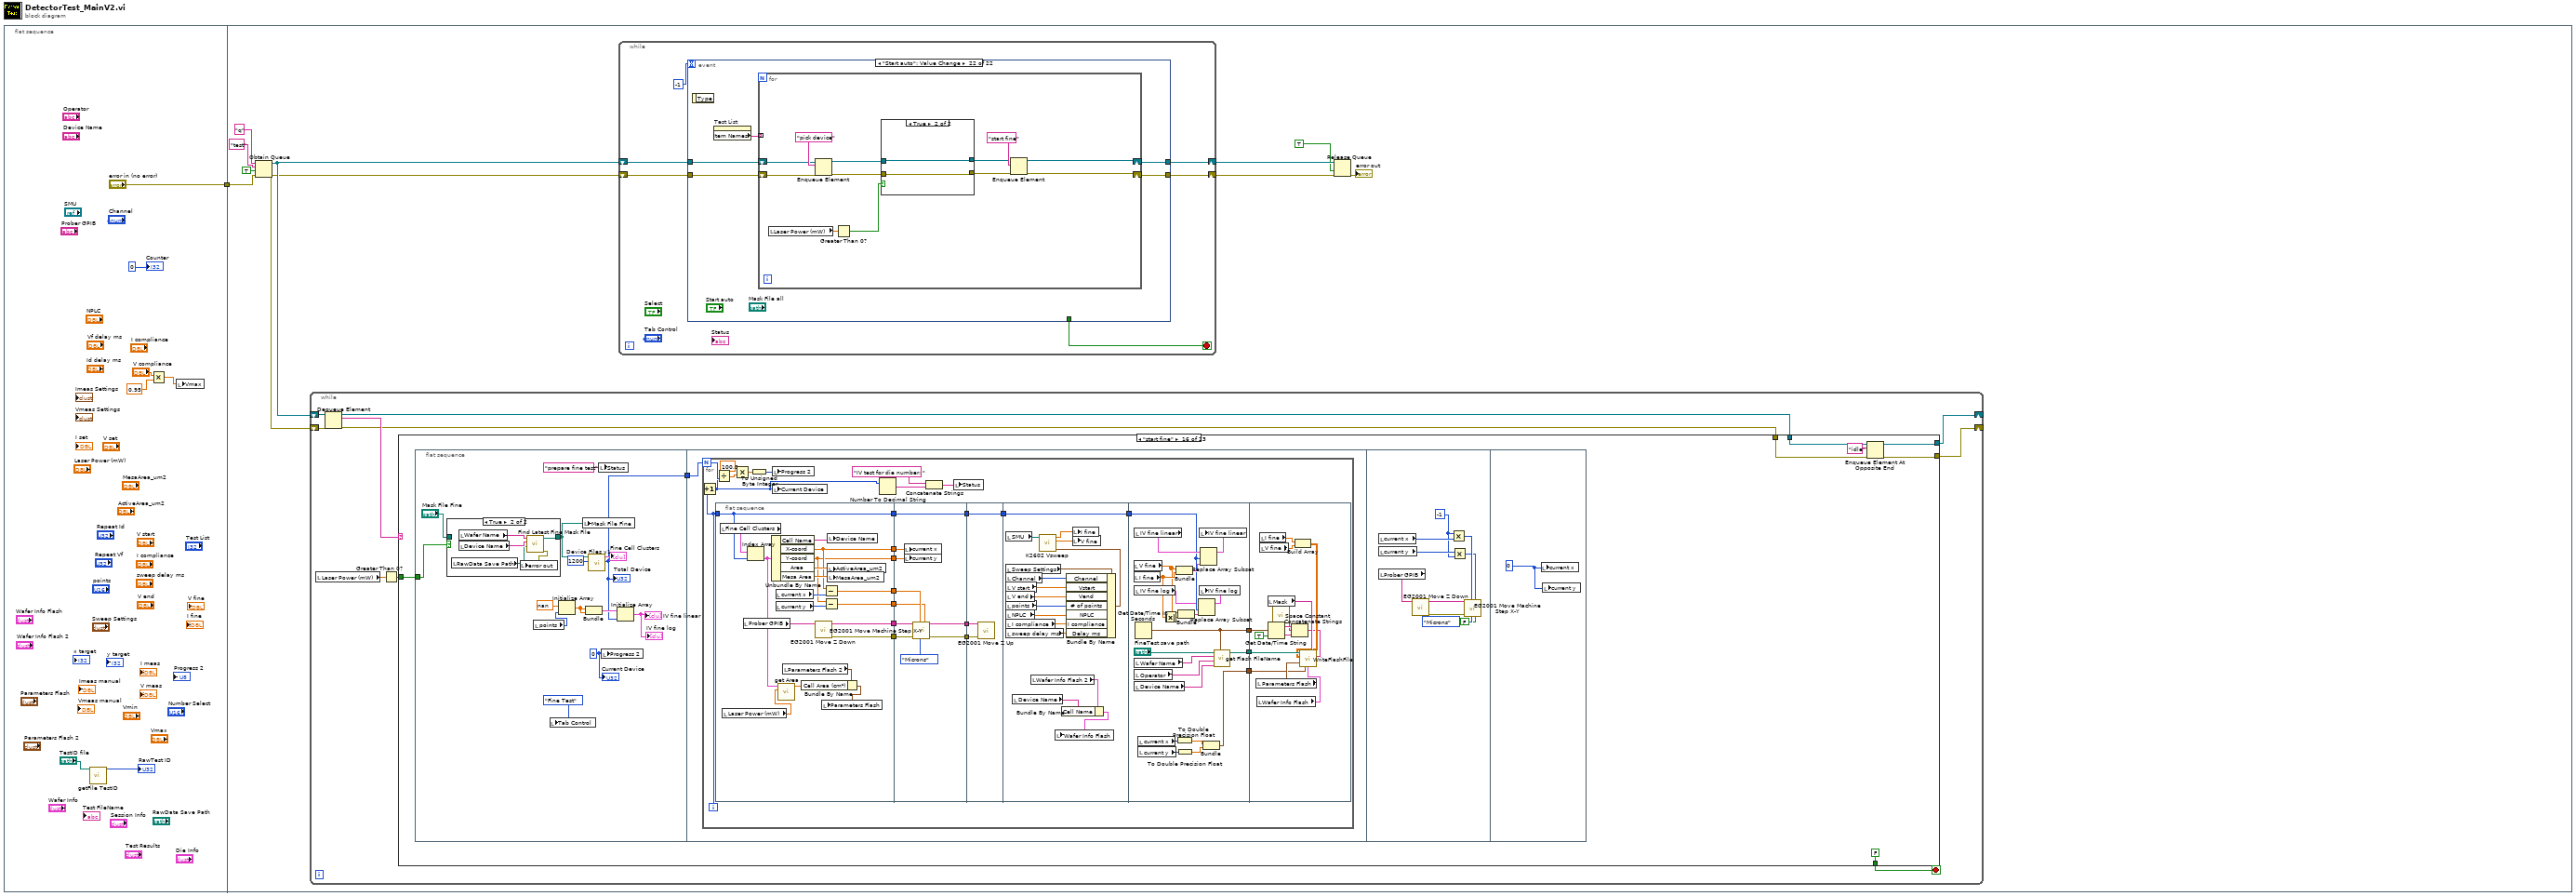
[diagram p0: block diagram]
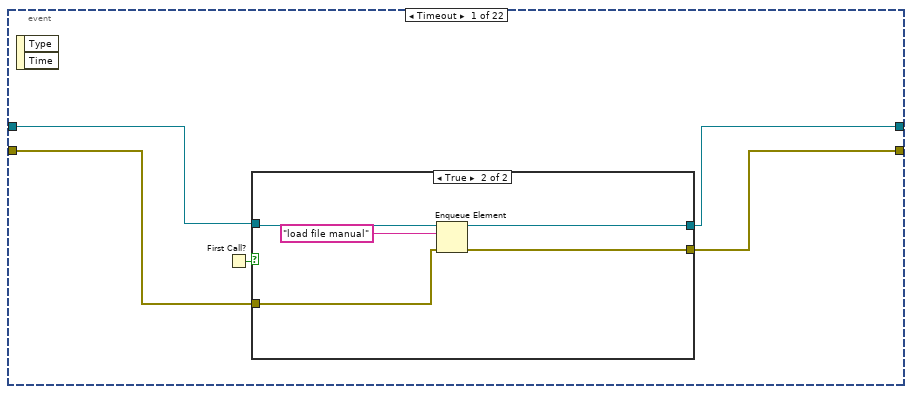
[diagram p2: hidden frame]
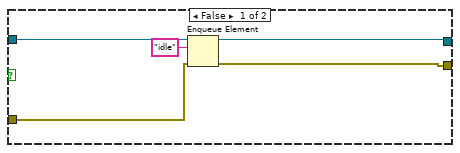
[diagram p3: hidden frame]
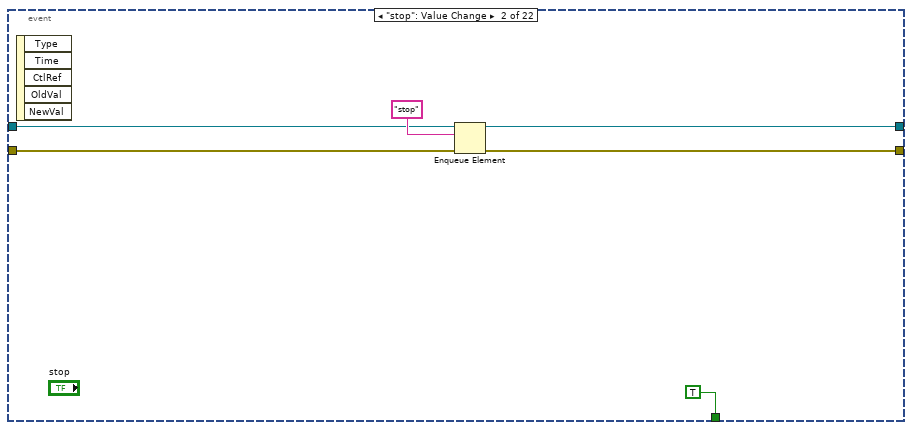
[diagram p4: hidden frame]
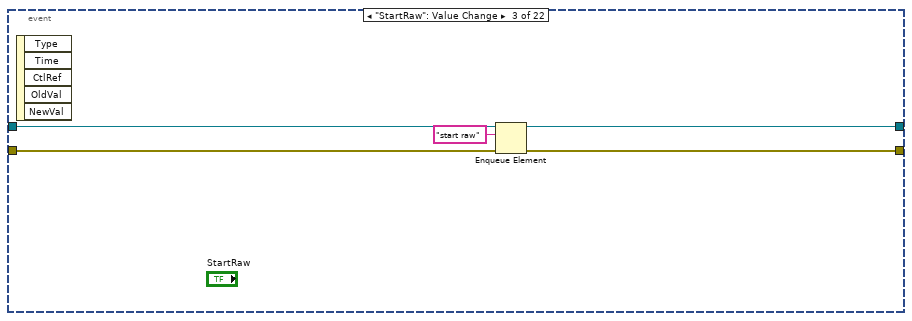
[diagram p5: hidden frame]
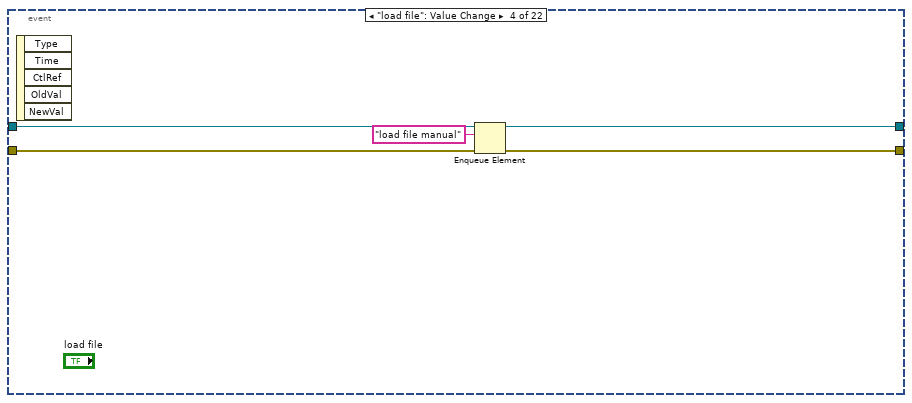
[diagram p6: hidden frame]
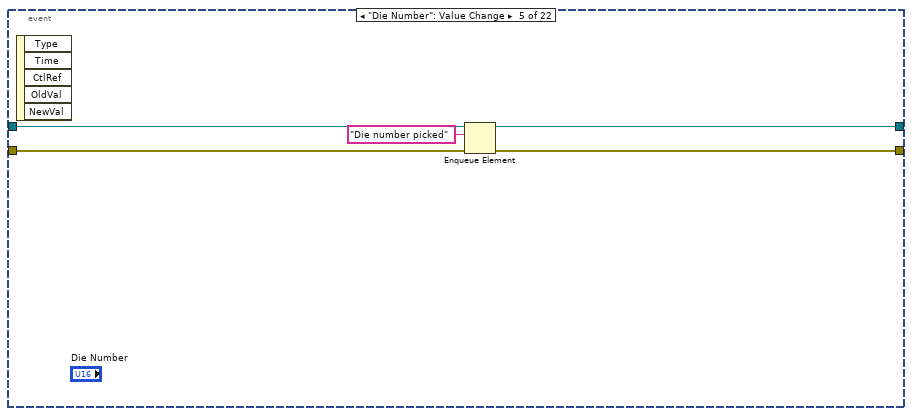
[diagram p7: hidden frame]
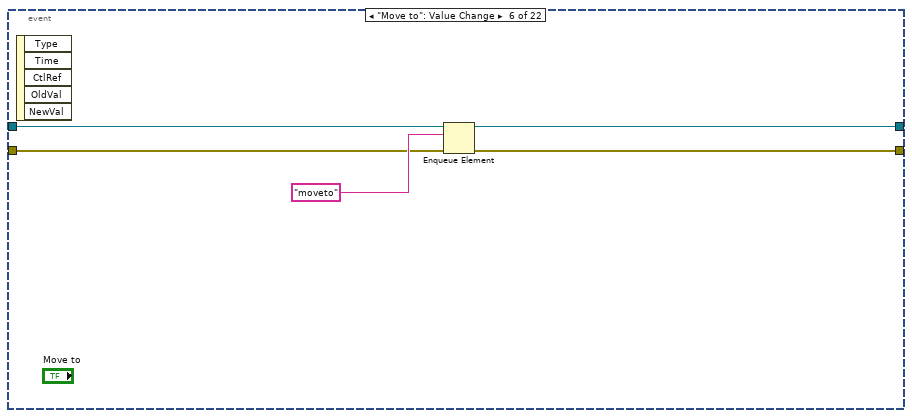
[diagram p8: hidden frame]
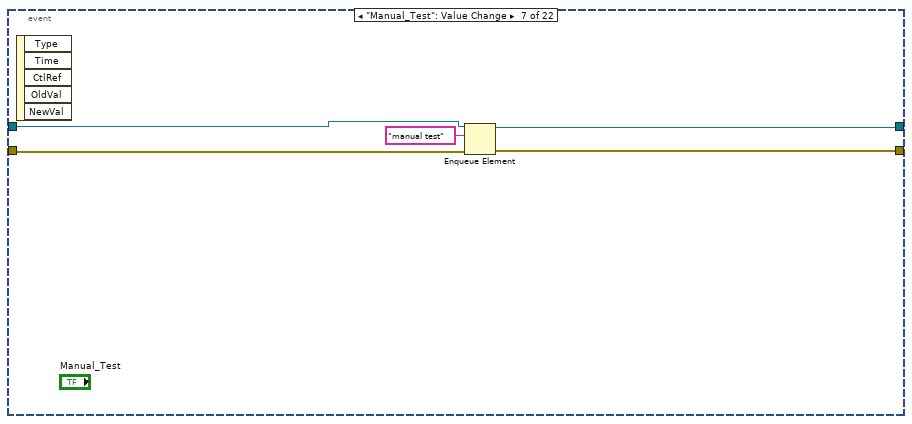
[diagram p9: hidden frame]
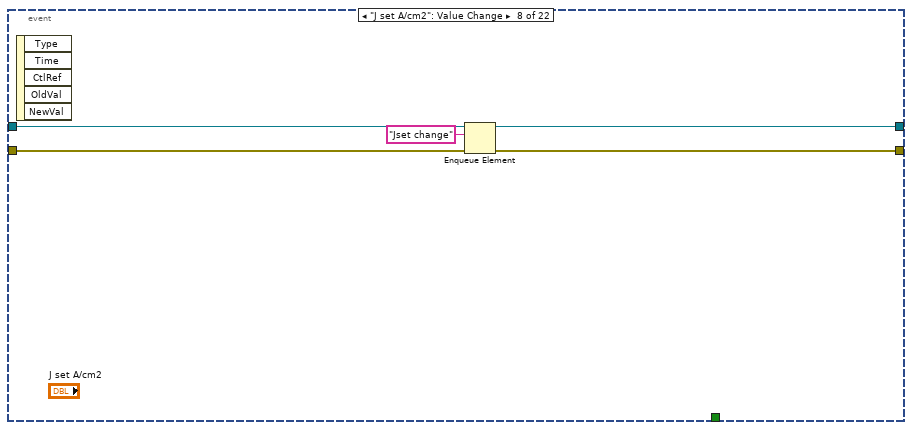
[diagram p10: hidden frame]
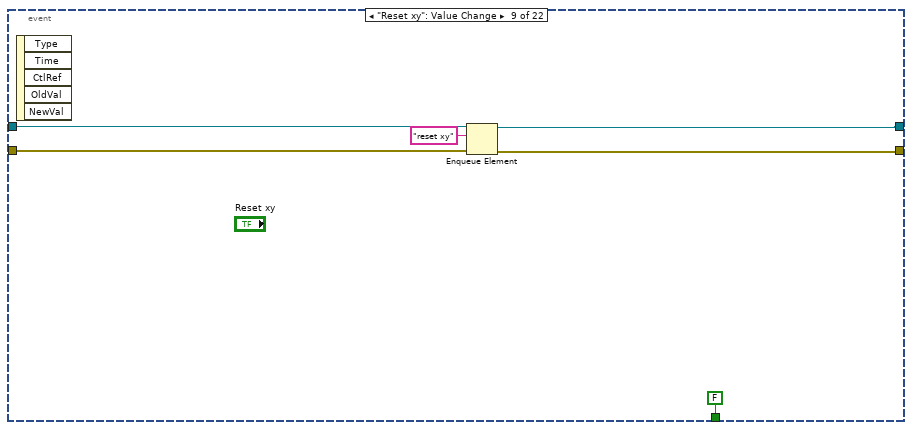
[diagram p11: hidden frame]
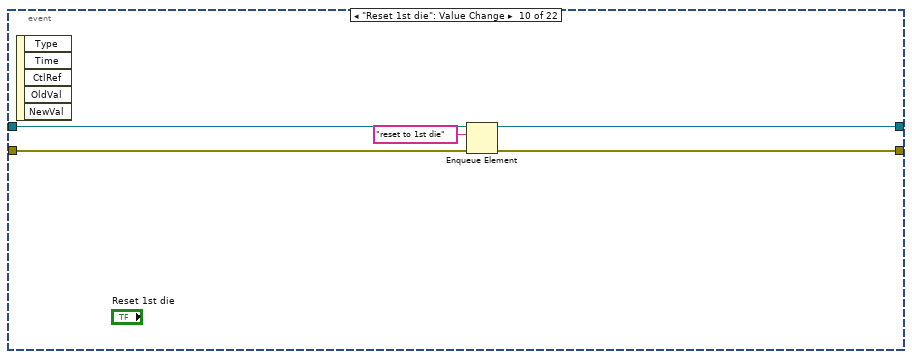
[diagram p12: hidden frame]
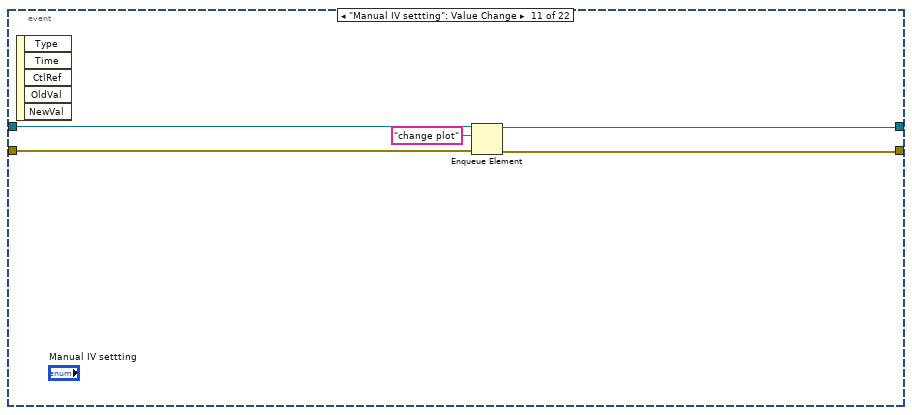
[diagram p13: hidden frame]
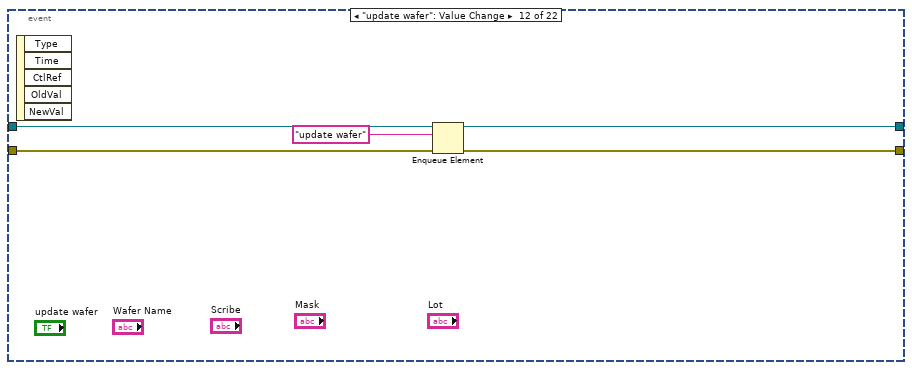
[diagram p14: hidden frame]
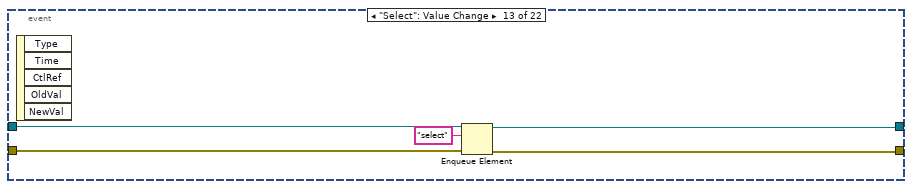
[diagram p15: hidden frame]
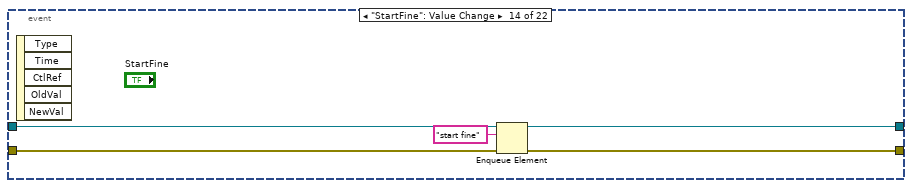
[diagram p16: hidden frame]
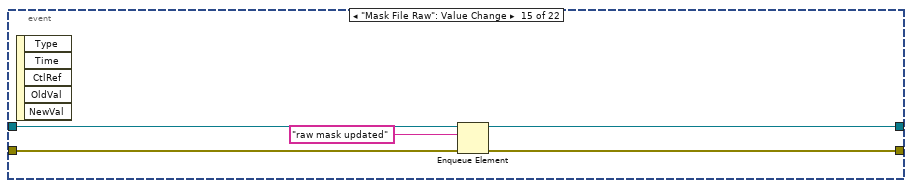
[diagram p17: hidden frame]
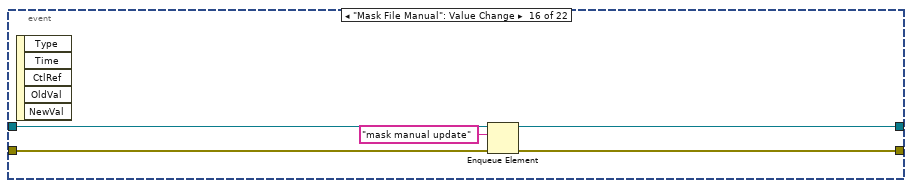
[diagram p18: hidden frame]
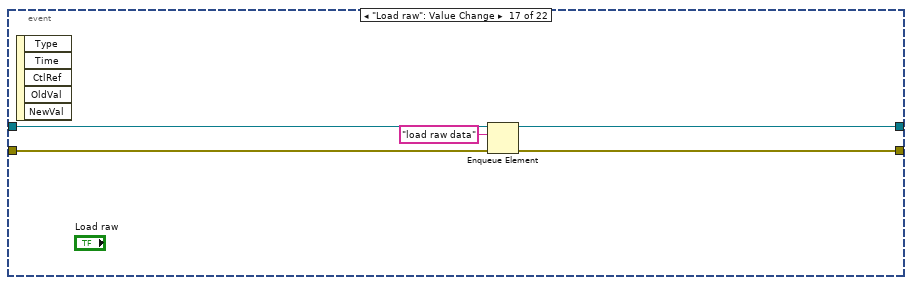
[diagram p19: hidden frame]
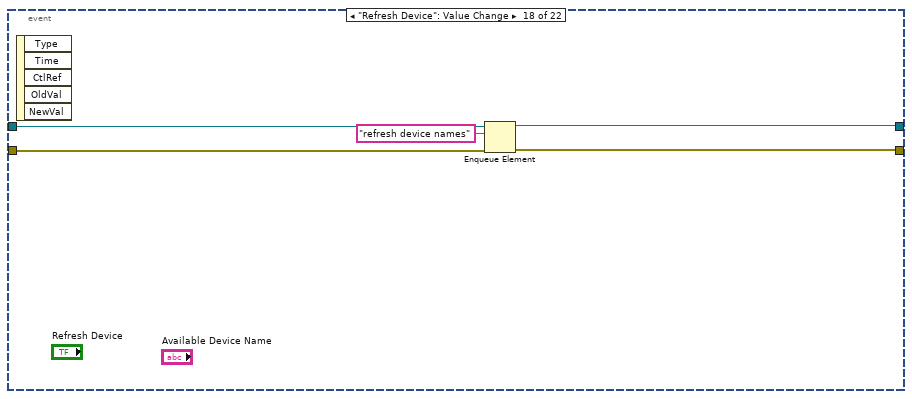
[diagram p20: hidden frame]
diagram:
  n1 = flat-sequence {
    tunnel: ["error in (no error)"] -> w1
    tunnel: w1 -> [w15]
    frame #0 {
      n2 = call "getFile TestID.vi"("Path"="TestID file") -> ("TestID"=→"RawTest ID":u32)  [unwired: 9 in, 1 out]
      n3 = Multiply(x="V compliance", y=0.95) -> (x*y=w3:dbl)
      n4 = local write "Vmax"(w3) -> ()
      "Counter" <- u32 0 ("Counter")
    }
    frame #1 {
      n5 = Obtain Queue(name (unnamed)="q", element data type="test" ("name (unnamed)"), create if not found? (T)=TRUE, error in (no error)=w15) -> (queue out=w17:refnum<queue>, error out=w16:errorcluster)  [unwired: 1 in, 1 out]
      n6 = while {
        shift-right: [w176] -> _
        shift-left: w17 -> [w173]
        shift-right: [w175] -> _
        shift-left: w16 -> [w172]
        stop <- w178 stop-if-true
        n7 = local read "Laser Power (mW)"() -> (w170:dbl)
        n8 = Dequeue Element(queue=w173, error in (no error)=w172) -> (queue out=w171:refnum<queue>, element=w177:string, error out=w174:errorcluster)  [unwired: 1 in, 1 out]
        n9 = Greater Than 0?(x=w170) -> (x > 0?=w169:bool)
        n10 = case shown="\"start fine\"" w177 {
          tunnel: [FALSE TRUE FALSE FALSE FALSE FALSE FALSE FALSE FALSE FALSE FALSE FALSE FALSE FALSE FALSE FALSE FALSE FALSE FALSE FALSE FALSE FALSE FALSE] -> w178
          tunnel: w174 -> [w180 w183 w188 w350 w361 w372 w403 w427 w438 w468 w548 w558 w565 w580 w617 w655 w805 w816 w825 w833 w841 w849 w857]
          tunnel: [w180 w183 w189 w351 w358 w369 w406 w428 w441 w467 w553 w558 w564 w582 w619 w657 w807 w818 w827 w836 w843 w852 w856] -> w175
          tunnel: w171 -> [w179 w182 w191 w353 w360 w371 w404 w430 w443 w465 w555 w559 w563 w581 w618 w656 w806 w817 w826 w835 w842 w851 w859]
          tunnel: [w179 w182 w190 w352 w359 w370 w405 w429 w442 w466 w554 w559 w562 w583 w620 w658 w808 w819 w828 w837 w844 w853 w858] -> w176
          tunnel: w169 -> [_ _ _ _ _ _ _ _ _ _ _ _ _ _ _ w651 _ _ _ _ _ _ _]
          frame "False", Default {
          }
          frame "stop" {
          }
          frame "start raw" {
            n11 = flat-sequence {
              tunnel: [w203] -> w187
              tunnel: w187 -> [w233]
              tunnel: [w233] -> w186
              tunnel: [w223] -> w185
              tunnel: w186 -> [w235]
              tunnel: w185 -> [w234]
              frame #0 {
                n12 = local read "Wafer Name"() -> (w201:string)
                n13 = local read "RawTest ID"() -> (w206:u32)
                n14 = local write "Tab Control"(T12."Raw Test" ("Tab Control")) -> ()
                n15 = local read "Scribe"() -> (w200:string)
                n16 = local read "Mask"() -> (w199:string)
                n17 = local read "Lot"() -> (w198:string)
                n18 = call "Device Files v1.vi"("Rows"=1200, "Mask file path"="Mask File Raw") -> ("size(s)"=w203:i32, "Array of Cell Clusters"=→"Array of Cell Data Clusters":T3)  [unwired: 6 in, 2 out]
                "Total Device" <- w203
                n19 = Increment(x=w206) -> (x+1=w205:u32)
                n20 = Bundle By Name(cluster="Wafer Info 2", "Wafer Name"=w201, "Scribe"=w200, "Mask"=w199, "Lot"=w198) -> (w202:T7)
                n21 = local write "Status"("Prepare raw test" ("Status")) -> ()
                n22 = Initialize Array(nan ("element"), w203) -> (w196:dbl[])
                n23 = local write "RawTest ID"(w205) -> ()
                n24 = Bundle(w196, w196) -> (→"Selected Data":cluster{dbl[], dbl[]})  [unwired: 1 in]
                n25 = local write "Wafer Info"(w202) -> ()
                n26 = local write "V meas"(w196) -> ()
                n27 = local write "I meas"(w196) -> ()
                "Progress" <- u8 0 ("Progress")
              }
              frame #1 {
                n28 = local read "Laser Power (mW)"() -> (w214:dbl)
                n29 = local read "V compliance"() -> (w215:dbl)
                n30 = local read "RawData Save Path"() -> (w227:path)
                n31 = local read "I compliance"() -> (w218:dbl)
                n32 = local read "RawTest ID"() -> (w213:u32)
                n33 = local read "Array of Cell Data Clusters"() -> (w232:T11)
                n34 = local read "Operator"() -> (w212:string)
                n35 = local read "J set A/cm2"() -> (w217:dbl)
                n36 = local read "Wafer Name"() -> (w229:string)
                n37 = local read "V set"() -> (w219:dbl)
                n38 = local read "I set"() -> (w216:dbl)
                n39 = Index Array(array=w232, index=0) -> (element=w230:T14)
                n40 = Unbundle By Name(w230) -> ("Cell Name"=w228:string)
                n41 = call "get RawTest filename.vi"("Device Name"=w228, "Wafer Name"=w229) -> ("current time"=w220:timestamp, "FileName"=w226:string)  [unwired: 8 in]
                n42 = Build Path(base path=w227, name or relative path=w226) -> (appended path=w225:path)
                n43 = local write "Test FileName"(w226) -> ()
                n44 = Bundle By Name(cluster="Session Info 2", "V set"=w219, "I compliance"=w218, "J set"=w217, "I set"=w216, "V compliance"=w215, "Laser Power (mW)"=w214, "TestID"=w213, "Session Time"=w220, "Operator"=w212) -> (w221:T5)
                n45 = call "writeFile RawTestHead.vi"("Name Array"="Name Array", "Path"=w225) -> ("Path out"=w223:path)  [unwired: 9 in]
                "RawData file" <- w223
                n46 = local write "Session Info"(w221) -> ()
              }
              frame #2 {
                n47 = for {
                  N: w235 -> [w248]
                  tunnel: w234 -> [w236]
                  i -> [w237]
                  n48 = flat-sequence {
                    tunnel: [w283] -> w258
                    tunnel: [w282] -> w257
                    tunnel: w237 -> [w276]
                    tunnel: [w278] -> w252
                    tunnel: [w277] -> w251
                    tunnel: [w260] -> w250
                    tunnel: [w259] -> w249
                    tunnel: w258 -> [w284]
                    tunnel: w257 -> [w292]
                    tunnel: [w291] -> w256
                    tunnel: [w290] -> w255
                    tunnel: w252 -> [w288]
                    tunnel: w251 -> [w287]
                    tunnel: w250 -> [w286]
                    tunnel: w249 -> [w285]
                    tunnel: w256 -> [w295]
                    tunnel: w255 -> [w294]
                    tunnel: [w305] -> w254
                    tunnel: [w304] -> w253
                    tunnel: w254 -> [w308]
                    tunnel: w253 -> [w316]
                    tunnel: [w308] -> w239
                    tunnel: [w309] -> w238
                    tunnel: w239 -> [w327]
                    tunnel: w238 -> [w326]
                    tunnel: w237 -> [w333]
                    tunnel: w236 -> [w324]
                    frame #0 {
                      n49 = local read "Array of Cell Data Clusters"() -> (w280:T11)
                      n50 = local read "Device Name"() -> (w263:string)
                      n51 = Increment(x=w276) -> (x+1=→"Current Device":i32)
                      n52 = local read "Laser Power (mW)"() -> (w272:dbl)
                      n53 = Index Array(array=w280, index=w276) -> (element=w273:T14)
                      n54 = local read "Prober GPIB"() -> (w274:string)
                      n55 = Unbundle By Name(w273) -> ("X-coord"=w260:dbl, "Y-coord"=w259:dbl, "Area"=w261:dbl, "Meas Area"=w262:dbl, "Cell Name"=w266:string)
                      n56 = Bundle By Name(cluster="Die Info 2", "Device Name"=w263, "ActiveArea_um2"=w261, "MesaArea_um2"=w262, "x"=w260, "y"=w259) -> (w264:T6)
                      n57 = call "get Area.vi"("Laser"=w272, "Cell Data Cluster"=w273) -> ("Area"=w270:dbl)  [unwired: 9 in]
                      n58 = local read "J set A/cm2"() -> (w268:dbl)
                      n59 = local write "ActiveArea_um2"(w261) -> ()
                      n60 = local write "MesaArea_um2"(w262) -> ()
                      n61 = local write "Device Name"(w266) -> ()
                      n62 = Divide(x=w270, y=100000000.0) -> (x/y=w269:dbl)
                      n63 = local read "current y"() -> (w279:i32)
                      n64 = call "EG2001 Move Z Down.vi"("GPIB Address"=w274) -> ("Error Out"=w282:errorcluster, "GPIB Address Out"=w283:string)  [unwired: 9 in]
                      n65 = local read "current x"() -> (w281:i32)
                      n66 = local write "Die Info"(w264) -> ()
                      n67 = Multiply(x=w268, y=w269) -> (x*y=w267:dbl)
                      n68 = local write "I set"(w267) -> ()
                      n69 = Subtract(x=w260, y=w281) -> (x-y=w278:dbl)
                      n70 = Subtract(x=w259, y=w279) -> (x-y=w277:dbl)
                    }
                    frame #1 {
                      n71 = local write "current x"(w286) -> ()
                      n72 = local write "current y"(w285) -> ()
                      n73 = call "EG2001 Move Machine Step X-Y.vi"("Flip X Coordinates?"=FALSE, "Y"=w287, "Steps/Microns"=enum32{"Steps", "Microns"}."Microns", "X"=w288, "error in (no error)"=w292, "GPIB Address"=w284) -> ("Error Out"=w290:errorcluster, "GPIB Address Out"=w291:string)  [unwired: 4 in]
                    }
                    frame #2 {
                      n74 = call "EG2001 Move Z Up.vi"("error in (no error)"=w294, "GPIB Address"=w295) -> ()  [unwired: 10 out]
                    }
                    frame #3 {
                      n75 = local read "SMU"() -> (w304:refnum<visa-resource-name>)
                      n76 = local read "Imeas Settings"() -> (w303:T10)
                      n77 = local read "Channel"() -> (w302:enum32{"Channel A", "Channel B"})
                      n78 = local read "V set"() -> (w296:dbl)
                      n79 = local read "NPLC"() -> (w301:dbl)
                      n80 = local read "I compliance"() -> (w300:dbl)
                      n81 = local read "Repeat Id"() -> (w299:u32)
                      n82 = local read "Id delay ms"() -> (w298:dbl)
                      n83 = Bundle By Name(cluster=w303, "Channel"=w302, "Vset"=w296, "NPLC"=w301, "I compliance"=w300, "Repeat time"=w299, "Delay ms"=w298) -> (w297:T10)
                      n84 = call "K2602 setVmeasI.vi"("Settings"=w297, "SMU"=w304) -> ("Iavg"=w305:dbl)  [unwired: 6 in, 3 out]
                    }
                    frame #4 {
                      n85 = local read "Vmeas Settings"() -> (w315:T9)
                      n86 = local read "Channel"() -> (w313:enum32{"Channel A", "Channel B"})
                      n87 = local read "NPLC"() -> (w307:dbl)
                      n88 = local read "V compliance"() -> (w312:dbl)
                      n89 = local read "Repeat Vf"() -> (w311:u32)
                      n90 = local read "Vf delay ms"() -> (w310:dbl)
                      n91 = local read "I set"() -> (w306:dbl)
                      n92 = Bundle By Name(cluster=w315, "Channel"=w313, "Iset"=w306, "NPLC"=w307, "V compliance"=w312, "Repeat time"=w311, "Delay ms"=w310) -> (w314:T9)
                      n93 = call "K2602 setImeasV.vi"("Settings"=w314, "SMU"=w316) -> ("Vavg"=w309:dbl)  [unwired: 6 in, 3 out]
                    }
                    frame #5 {
                      n94 = local read "I meas"() -> (w335:dbl[])
                      n95 = local read "V meas"() -> (w334:dbl[])
                      n96 = Get Date/Time In Seconds() -> (seconds since 1Jan1904=w325:timestamp)
                      n97 = Replace Array Subset(array=w335, new element=w327, index=w333) -> (w330:dbl[])
                      n98 = Replace Array Subset(array=w334, new element=w326, index=w333) -> (w329:dbl[])
                      n99 = call <vilib>:"Histogram.vi"("X"=w329) -> ("Histogram Graph"=→"Vforward hist":T13)  [unwired: 7 in, 3 out]
                      n100 = local read "Selected Data"() -> (w318:cluster{dbl[], dbl[]})
                      n101 = local write "V meas"(w329) -> ()
                      n102 = local write "I meas"(w330) -> ()
                      n103 = Bundle("V meas"=w329, "I meas"=w330) -> (w319:cluster{"V meas":dbl[], "I meas":dbl[]})  [unwired: 1 in]
                      n104 = Bundle By Name(cluster="Test Results 2", "I meas"=w327, "V meas"=w326, "Time"=w325) -> (w323:T4)
                      n105 = call <vilib>:"Histogram.vi"("X"=w330) -> ("Histogram Graph"=→"Idark hist":T13)  [unwired: 7 in, 3 out]
                      n106 = local write "Test Results"(w323) -> ()
                      n107 = local read "Session Info"() -> (w320:T5)
                      n108 = local read "Die Info"() -> (w321:T6)
                      n109 = local read "Wafer Info"() -> (w322:T7)
                      n110 = Build Array(w319, w318) -> (→"Spec Plot":cluster{"V meas":dbl[], "I meas":dbl[]}[])
                      n111 = call "writeFile RawTestData.vi"("Test Results"=w323, "Session Info"=w320, "Die Info"=w321, "Wafer Info"=w322, "Path"=w324) -> ()  [unwired: 6 in, 1 out]
                    }
                  }
                  n112 = Divide(x=w237, y=w248) -> (x/y=w246:dbl)
                  n113 = Multiply(x=w246, y=100.0) -> (x*y=w244:dbl)
                  n114 = To Unsigned Byte Integer(number=w244) -> (unsigned 8bit integer=w247:u8)
                  n115 = local write "Progress"(w247) -> ()
                  n116 = Increment(x=w237) -> (x+1=w240:i32)
                  n117 = Number To Decimal String(number=w240) -> (decimal integer string=w242:string)  [unwired: 1 in]
                  n118 = Concatenate Strings("Raw Test for die number:" ("string"), w242) -> (w243:string)
                  n119 = local write "Status"(w243) -> ()
                }
              }
              frame #3 {
                w340 = -1
                n120 = local read "TestID file"() -> (w336:path)
                n121 = local read "RawTest ID"() -> (w337:u32)
                n122 = local read "current x"() -> (w342:i32)
                n123 = local read "current y"() -> (w341:i32)
                n124 = local read "Prober GPIB"() -> (w347:string)
                n125 = call "EG2001 Move Z Down.vi"("GPIB Address"=w347) -> ("Error Out"=w346:errorcluster, "GPIB Address Out"=w345:string)  [unwired: 9 in]
                n126 = call "writeFile TestID.vi"("TestID"=w337, "Path"=w336) -> ()  [unwired: 10 in]
                n127 = Multiply(x=w340, y=w342) -> (x*y=w339:i32)
                n128 = Multiply(x=w340, y=w341) -> (x*y=w338:i32)
                n129 = call "EG2001 Move Machine Step X-Y.vi"("Flip X Coordinates?"=FALSE, "Y"=w338, "Steps/Microns"=enum32{"Steps", "Microns"}."Microns", "X"=w339, "error in (no error)"=w346, "GPIB Address"=w345) -> ()  [unwired: 4 in, 2 out]
              }
              frame #4 {
                w348 = 0
                n130 = local write "current x"(w348) -> ()
                n131 = local write "current y"(w348) -> ()
              }
            }
            n132 = Enqueue Element At Opposite End(queue=w191, element="idle", error in (no error)=w188) -> (queue out=w190:refnum<queue>, error out=w189:errorcluster)  [unwired: 1 in, 1 out]
          }
          frame "reset xy" {
            n133 = local read "Prober GPIB"() -> (w349:string)
            n134 = call "EG2001 Move First.vi"("GPIB Address"=w349) -> ()  [unwired: 9 in, 2 out]
            n135 = Enqueue Element At Opposite End(queue=w353, element="idle", error in (no error)=w350) -> (queue out=w352:refnum<queue>, error out=w351:errorcluster)  [unwired: 1 in, 1 out]
            "current x" <- u32 0 ("current x")
            "current y" <- u32 0 ("current y")
          }
          frame "reset to 1st die" {
            n136 = local read "Array of Cell Data Clusters"() -> (w367:T11)
            n137 = Index Array(array=w367, index=0) -> (element=w365:T14)
            n138 = Unbundle By Name(w365) -> ("X-coord"=w364:dbl, "Y-coord"=w363:dbl)
            n139 = local write "current x"(w364) -> ()
            n140 = local write "current y"(w363) -> ()
            n141 = Enqueue Element At Opposite End(queue=w360, element="idle", error in (no error)=w361) -> (queue out=w359:refnum<queue>, error out=w358:errorcluster)  [unwired: 1 in, 1 out]
          }
          frame "load file manual" {
            n142 = flat-sequence {
              tunnel: [w379] -> w374
              tunnel: w374 -> [w383]
              frame #0 {
                n143 = call "Device Files v1.vi"("Rows"=1200, "Mask file path"="Mask File Manual") -> ("Mask Name"=w380:string, "size(s)"=w379:i32, "Array of Cell Clusters"=w376:T3)  [unwired: 6 in, 1 out]
                n144 = local write "Array of Cell Data Clusters"(w376) -> ()
                n145 = local write "Status"("Loading mask file" ("Status")) -> ()
                n146 = local write "Mask"(w380) -> ()
              }
              frame #1 {
                n147 = for {
                  N: w383 -> [_]
                  tunnel: [w384] -> w382 mode=indexing
                  i -> [w385]
                  n148 = Number To Decimal String(number=w385) -> (decimal integer string=w384:string)  [unwired: 1 in]
                }
                n149 = property on="Die Number" class="Ring (strict)"("Strings []"=w382) -> ()  [unwired: 2 in, 2 out]
              }
              frame #2 {
                n150 = local read "Array of Cell Data Clusters"() -> (w393:T11)
                n151 = local read "Die Number"() -> (w392:u16)
                n152 = Index Array(array=w393, index=w392) -> (element=w391:T14)
                n153 = Unbundle By Name(w391) -> ("Cell Name"=w386:string, "X-coord"=w389:dbl, "Y-coord"=w390:dbl, "Area"=w388:dbl, "Meas Area"=w387:dbl)
                n154 = local write "Device Name"(w386) -> ()
                n155 = local write "x target"(w389) -> ()
                n156 = local write "y target"(w390) -> ()
                n157 = local write "ActiveArea_um2"(w388) -> ()
                n158 = local write "MesaArea_um2"(w387) -> ()
              }
              frame #3 {
                n159 = local read "Laser Power (mW)"() -> (w396:dbl)
                n160 = Equal To 0?(x=w396) -> (x = 0?=w395:bool)
                n161 = case shown="True" w395 {
                  tunnel: [w401 w402] -> w394
                  frame False {
                    n162 = local read "ActiveArea_um2"() -> (w401:dbl)
                  }
                  frame True {
                    n163 = local read "MesaArea_um2"() -> (w402:dbl)
                  }
                }
                n164 = local read "J set A/cm2"() -> (w399:dbl)
                n165 = Divide(x=w394, y=100000000.0) -> (x/y=w398:dbl)
                n166 = Multiply(x=w398, y=w399) -> (x*y=w400:dbl)
                n167 = local write "I set"(w400) -> ()
              }
            }
            n168 = Enqueue Element At Opposite End(queue=w371, element="idle", error in (no error)=w372) -> (queue out=w370:refnum<queue>, error out=w369:errorcluster)  [unwired: 1 in, 1 out]
          }
          frame "Die number picked" {
            n169 = flat-sequence {
              frame #0 {
                n170 = local read "Array of Cell Data Clusters"() -> (w417:T11)
                n171 = local read "Die Number"() -> (w416:u16)
                n172 = Index Array(array=w417, index=w416) -> (element=w415:T14)
                n173 = Unbundle By Name(w415) -> ("Cell Name"=w412:string, "X-coord"=w414:dbl, "Y-coord"=w413:dbl, "Area"=w411:dbl, "Meas Area"=w410:dbl)
                n174 = local write "Device Name"(w412) -> ()
                n175 = local write "x target"(w414) -> ()
                n176 = local write "y target"(w413) -> ()
                n177 = local write "ActiveArea_um2"(w411) -> ()
                n178 = local write "MesaArea_um2"(w410) -> ()
              }
              frame #1 {
                n179 = local read "Laser Power (mW)"() -> (w420:dbl)
                n180 = Equal To 0?(x=w420) -> (x = 0?=w419:bool)
                n181 = case shown="True" w419 {
                  tunnel: [w425 w426] -> w418
                  frame False {
                    n182 = local read "ActiveArea_um2"() -> (w425:dbl)
                  }
                  frame True {
                    n183 = local read "MesaArea_um2"() -> (w426:dbl)
                  }
                }
                n184 = local read "J set A/cm2"() -> (w423:dbl)
                n185 = Divide(x=w418, y=100000000.0) -> (x/y=w422:dbl)
                n186 = Multiply(x=w422, y=w423) -> (x*y=w424:dbl)
                n187 = local write "I set"(w424) -> ()
              }
            }
            n188 = local write "Status"("Changing Die" ("Status")) -> ()
            n189 = Enqueue Element At Opposite End(queue=w404, element="idle", error in (no error)=w403) -> (queue out=w405:refnum<queue>, error out=w406:errorcluster)  [unwired: 1 in, 1 out]
          }
          frame "Jset change" {
            n190 = local read "ActiveArea_um2"() -> (w436:dbl)
            n191 = local read "J set A/cm2"() -> (w433:dbl)
            n192 = Divide(x=w436, y=100000000.0) -> (x/y=w434:dbl)
            n193 = Multiply(x=w434, y=w433) -> (x*y=w432:dbl)
            n194 = local write "I set"(w432) -> ()
            n195 = Enqueue Element At Opposite End(queue=w430, element="idle", error in (no error)=w427) -> (queue out=w429:refnum<queue>, error out=w428:errorcluster)  [unwired: 1 in, 1 out]
          }
          frame "moveto" {
            n196 = flat-sequence {
              tunnel: [w449] -> w440
              tunnel: [w448] -> w439
              tunnel: w440 -> [w454]
              tunnel: w439 -> [w453]
              frame #0 {
                n197 = local read "Prober GPIB"() -> (w447:string)
                n198 = local write "Status"("Probe up" ("Status")) -> ()
                n199 = call "EG2001 Move Z Down.vi"("GPIB Address"=w447) -> ("Error Out"=w448:errorcluster, "GPIB Address Out"=w449:string)  [unwired: 9 in]
              }
              frame #1 {
                n200 = local read "y target"() -> (w458:i32)
                n201 = local read "x target"() -> (w460:i32)
                n202 = local read "current x"() -> (w459:i32)
                n203 = local read "current y"() -> (w457:i32)
                n204 = local write "Status"("Moving Probe" ("Status")) -> ()
                n205 = Subtract(x=w460, y=w459) -> (x-y=w456:i32)
                n206 = Subtract(x=w458, y=w457) -> (x-y=w455:i32)
                n207 = call "EG2001 Move Machine Step X-Y.vi"("Flip X Coordinates?"=FALSE, "Y"=w455, "Steps/Microns"=enum32{"Steps", "Microns"}."Microns", "X"=w456, "error in (no error)"=w453, "GPIB Address"=w454) -> ()  [unwired: 4 in, 2 out]
              }
              frame #2 {
                n208 = local read "x target"() -> (w463:i32)
                n209 = local read "y target"() -> (w462:i32)
                n210 = local write "current y"(w462) -> ()
                n211 = local write "current x"(w463) -> ()
                n212 = local write "Status"("Done" ("Status")) -> ()
              }
            }
            n213 = Enqueue Element At Opposite End(queue=w443, element="idle", error in (no error)=w438) -> (queue out=w442:refnum<queue>, error out=w441:errorcluster)  [unwired: 1 in, 1 out]
          }
          frame "manual test" {
            n214 = flat-sequence {
              tunnel: [w481] -> w478
              tunnel: [w480] -> w477
              tunnel: [w486] -> w476
              tunnel: [w485] -> w475
              tunnel: w478 -> [w485]
              tunnel: [w484] -> w474
              tunnel: w477 -> [w484]
              tunnel: w476 -> [w510]
              tunnel: [w510] -> w473
              tunnel: [w500] -> w472
              tunnel: w475 -> [w500]
              tunnel: [w499] -> w471
              tunnel: w474 -> [w499]
              tunnel: w473 -> [w523]
              tunnel: [w513] -> w470
              tunnel: w472 -> [w513]
              tunnel: [w512] -> w469
              tunnel: w471 -> [w512]
              tunnel: w470 -> [w537]
              tunnel: w469 -> [w536]
              frame #0 {
                n215 = local read "Prober GPIB"() -> (w482:string)
                n216 = call "EG2001 Move Z Up.vi"("GPIB Address"=w482) -> ("Error Out"=w480:errorcluster, "GPIB Address Out"=w481:string)  [unwired: 1 in, 8 out]
              }
              frame #1 {
                n217 = local read "SMU"() -> (w486:refnum<visa-resource-name>)
                n218 = local read "Sweep Settings"() -> (w497:T8)
                n219 = local read "Channel"() -> (w496:enum32{"Channel A", "Channel B"})
                n220 = local read "V start"() -> (w495:dbl)
                n221 = local read "V end"() -> (w494:dbl)
                n222 = local read "points"() -> (w493:u16)
                n223 = local read "NPLC"() -> (w492:dbl)
                n224 = local read "I compliance"() -> (w491:dbl)
                n225 = local read "sweep delay ms"() -> (w490:dbl)
                n226 = Bundle By Name(cluster=w497, "Channel"=w496, "Vstart"=w495, "Vend"=w494, "# of points"=w493, "NPLC"=w492, "I compliance"=w491, "Delay ms"=w490) -> (w489:T8)
                n227 = call "K2602 Vsweep.vi"("Settings"=w489, "SMU"=w486) -> ("V"=→"Varray manual":dbl[], "I"=→"Iarray manual":dbl[])  [unwired: 7 in, 1 out]
                n228 = local write "Status"("Sweeping IV Curve") -> ()
              }
              frame #2 {
                n229 = local read "Imeas Settings"() -> (w509:T10)
                n230 = local read "Channel"() -> (w506:enum32{"Channel A", "Channel B"})
                n231 = local read "V set"() -> (w505:dbl)
                n232 = local read "NPLC"() -> (w504:dbl)
                n233 = local read "I compliance"() -> (w503:dbl)
                n234 = local read "Repeat Id"() -> (w502:u32)
                n235 = local read "Id delay ms"() -> (w501:dbl)
                n236 = Bundle By Name(cluster=w509, "Channel"=w506, "Vset"=w505, "NPLC"=w504, "I compliance"=w503, "Repeat time"=w502, "Delay ms"=w501) -> (w508:T10)
                n237 = local write "Status"("Measuring I @ Vset") -> ()
                n238 = call "K2602 setVmeasI.vi"("Settings"=w508, "SMU"=w510) -> ("Iavg"=w507:dbl)  [unwired: 6 in, 3 out]
                n239 = local write "Imeas manual"(w507) -> ()
              }
              frame #3 {
                n240 = local read "Vmeas Settings"() -> (w521:T9)
                n241 = local read "Channel"() -> (w519:enum32{"Channel A", "Channel B"})
                n242 = local read "I set"() -> (w518:dbl)
                n243 = local read "NPLC"() -> (w517:dbl)
                n244 = local read "V compliance"() -> (w516:dbl)
                n245 = local read "Repeat Vf"() -> (w515:u32)
                n246 = local read "Vf delay ms"() -> (w514:dbl)
                n247 = Bundle By Name(cluster=w521, "Channel"=w519, "Iset"=w518, "NPLC"=w517, "V compliance"=w516, "Repeat time"=w515, "Delay ms"=w514) -> (w520:T9)
                n248 = local write "Status"("Measuring V @ Iset") -> ()
                n249 = call "K2602 setImeasV.vi"("Settings"=w520, "SMU"=w523) -> ("Vavg"=w522:dbl)  [unwired: 6 in, 3 out]
                n250 = local write "Vmeas manual"(w522) -> ()
              }
              frame #4 {
                n251 = local read "Imeas manual"() -> (w526:dbl)
                n252 = local read "Vmeas manual"() -> (w527:dbl)
                n253 = local read "points"() -> (w530:u16)
                n254 = local read "Varray manual"() -> (w529:dbl[])
                n255 = local read "Iarray manual"() -> (w528:dbl[])
                n256 = local read "V set"() -> (w525:dbl)
                n257 = local read "I set"() -> (w524:dbl)
                n258 = call "EG2001 Move Z Down.vi"("error in (no error)"=w536, "GPIB Address"=w537) -> ()  [unwired: 8 in, 2 out]
                n259 = local write "Status"("Done") -> ()
                n260 = local read "Manual IV settting"() -> (w535:enum32{"Linear plot", "Log plot"})
                n261 = call "get Plot.vi"("I set"=w524, "Imeas"=w526, "V set"=w525, "Vmeas"=w527, "Iarray"=w528, "Varray"=w529, "points"=w530) -> ("logplot"=w532:cluster{"Varray manual":dbl[], dbl[]}[], "Linearplot"=w531:T15)  [unwired: 3 in]
                "Manual Plot 0" <- w531
                "Manaul Plot 1" <- w532
                n262 = case shown="\"Linear plot\", Default" w535 {
                  tunnel: w531 -> [w540 _]
                  tunnel: [w540 w543] -> w534
                  tunnel: w532 -> [_ w543]
                  frame "Linear plot", Default {
                    n263 = property on="Manual IV" class="XYGraph (strict)"("YScale.Mapping Mode"=u8 0 ("Y Scale.Mapping Mode")) -> ()  [unwired: 2 in, 2 out]
                    n264 = property on="Manual IV" class="XYGraph (strict)"("YScale.NameLbl.Text"="Current (A)" ("X Scale.Name Label.Text")) -> ()  [unwired: 2 in, 2 out]
                  }
                  frame "Log plot" {
                    n265 = property on="Manual IV" class="XYGraph (strict)"("YScale.NameLbl.Text"="Abs(I)" ("Y Scale.Name Label.Text")) -> ()  [unwired: 2 in, 2 out]
                    n266 = property on="Manual IV" class="XYGraph (strict)"("YScale.Mapping Mode"=u8 1 ("Y Scale.Mapping Mode")) -> ()  [unwired: 2 in, 2 out]
                  }
                }
                "Manual IV" <- w534
              }
            }
            n267 = Enqueue Element At Opposite End(queue=w465, element="idle", error in (no error)=w468) -> (queue out=w466:refnum<queue>, error out=w467:errorcluster)  [unwired: 1 in, 1 out]
          }
          frame "update wafer" {
            n268 = local read "Wafer Name"() -> (w546:string)
            n269 = call "getDB Wafer Info.vi"("Wafer Name"=w546) -> ("WaferInfo"=w547:T16)  [unwired: 9 in, 1 out]
            n270 = Unbundle By Name(w547) -> ("WaferName"=w544:string, "Scribe"=w552:string, "Lot"=w551:string, "Mask"=w550:string)  [unwired: 1 out]
            n271 = local write "Scribe"(w552) -> ()
            n272 = local write "Lot"(w551) -> ()
            n273 = local write "Mask"(w550) -> ()
            n274 = Equal?(x=w546, y=w544) -> (x = y?=w545:bool)
            n275 = case shown="False" w545 {
              tunnel: w544 -> [w557 _]
              frame False {
                n276 = local write "Wafer Name"(w557) -> ()
              }
              frame True {
              }
            }
            n277 = Enqueue Element At Opposite End(queue=w555, element="idle", error in (no error)=w548) -> (queue out=w554:refnum<queue>, error out=w553:errorcluster)  [unwired: 1 in, 1 out]
          }
          frame "idle" {
            n278 = local write "Status"("idle" ("Status")) -> ()
          }
          frame "change plot" {
            n279 = local read "Manual IV settting"() -> (w569:enum32{"Linear plot", "Log plot"})
            n280 = case shown="\"Log plot\"" w569 {
              tunnel: [w572 w575] -> w568
              frame "Linear plot", Default {
                n281 = local read "Manual Plot 0"() -> (w572:cluster{"V manual":dbl[], "I manual":dbl[]}[])
                n282 = property on="Manual IV" class="XYGraph (strict)"("YScale.NameLbl.Text"="Current (A)" ("Y Scale.Name Label.Text")) -> ()  [unwired: 2 in, 2 out]
                n283 = property on="Manual IV" class="XYGraph (strict)"("YScale.Mapping Mode"=u8 0 ("Y Scale.Mapping Mode")) -> ()  [unwired: 2 in, 2 out]
              }
              frame "Log plot" {
                n284 = local read "Manaul Plot 1"() -> (w575:cluster{"V manual":dbl[], dbl[]}[])
                n285 = property on="Manual IV" class="XYGraph (strict)"("YScale.Mapping Mode"=u8 1 ("Y Scale.Mapping Mode")) -> ()  [unwired: 2 in, 2 out]
                n286 = property on="Manual IV" class="XYGraph (strict)"("YScale.NameLbl.Text"="Abs(I)" ("Y Scale.Name Label.Text")) -> ()  [unwired: 2 in, 2 out]
              }
            }
            n287 = local write "Manual IV"(w568) -> ()
            n288 = Enqueue Element At Opposite End(queue=w563, element="idle", error in (no error)=w565) -> (queue out=w562:refnum<queue>, error out=w564:errorcluster)  [unwired: 1 in, 1 out]
          }
          frame "select" {
            n289 = local read "I meas"() -> (w578:dbl[])
            n290 = Array Size(array=w578) -> (size(s)=w576:i32)
            n291 = Greater Than 0?(x=w576) -> (x > 0?=w577:bool)
            n292 = case shown="True" w577 {
              tunnel: w576 -> [_ w602]
              frame False {
              }
              frame True {
                n293 = local read "Laser Power (mW)"() -> (w586:dbl)
                n294 = local read "Number Select"() -> (w608:u16)
                n295 = local read "I meas"() -> (w593:dbl[])
                n296 = local read "V meas"() -> (w594:dbl[])
                n297 = local read "Vmin"() -> (w606:dbl)
                n298 = local read "Vmax"() -> (w607:dbl)
                n299 = local read "RawData Save Path"() -> (w604:path)
                n300 = local read "Mask File Raw"() -> (w609:path)
                n301 = Greater Than 0?(x=w586) -> (x > 0?=w585:bool)
                n302 = local read "Wafer Name"() -> (w610:string)
                n303 = Initialize Array(nan ("element"), w602) -> (w598:dbl[])
                n304 = call "select RawTestData.vi"("Light > 0?"=w585, "Number Select"=w608, "Vmax"=w607, "Vmin"=w606, "V meas"=w594, "I meas"=w593) -> ("Selected V"=w601:dbl[], "Selected I"=w599:dbl[], "Selected Index"=w587:dbl[])  [unwired: 2 in, 1 out]
                n305 = Replace Array Subset(array=w598, new element=w601, index=0) -> (w596:dbl[])
                n306 = Replace Array Subset(array=w598, new element=w599, index=0) -> (w595:dbl[])
                n307 = call "save FineMask.vi"("Selected Index"=w587, "RawData Save Path"=w604, "Text Add"=w610, "Mask File Raw"=w609) -> ("Output path"=w605:path)  [unwired: 7 in]
                n308 = local read "RawData file"() -> (w589:path)
                n309 = Bundle(w596, w595) -> (w591:cluster{dbl[], dbl[]})  [unwired: 1 in]
                n310 = Bundle("V meas"=w594, "I meas"=w593) -> (w592:cluster{"V meas":dbl[], "I meas":dbl[]})  [unwired: 1 in]
                n311 = local write "Mask File Fine"(w605) -> ()
                n312 = Build Array(w592, w591) -> (w590:cluster{"V meas":dbl[], "I meas":dbl[]}[])
                n313 = call "updatedFile RawTestSelect.vi"("Column Number"=u32 21, "Selected Index"=w587, "Path"=w589) -> ()  [unwired: 9 in]
                n314 = local write "Spec Plot"(w590) -> ()
              }
            }
            n315 = Enqueue Element At Opposite End(queue=w581, element="idle", error in (no error)=w580) -> (queue out=w583:refnum<queue>, error out=w582:errorcluster)  [unwired: 1 in, 1 out]
          }
          frame "load raw data" {
            n316 = local read "RawData Save Path"() -> (w613:path)
            n317 = call "File Dialog"("start path"=w613, "prompt"="Please pick a raw test data file", "pattern (all files)"="*.csv" ("pattern label")) -> ("selected path"=w612:path, "cancelled"=w616:bool)  [unwired: 9 in, 2 out]
            n318 = case shown="False" w616 {
              tunnel: w612 -> [_ w622]
              frame True {
              }
              frame False {
                n319 = call "read Raw.vi"("Path"=w622) -> ("Session Info"=w641:T17, "Die Info"=w650:T18, "Wafer Info"=w649:T7, "V"=w627:dbl[], "I"=w626:dbl[])  [unwired: 6 in]
                n320 = Array Size(array=w626) -> (size(s)=w632:i32)
                n321 = Strip Path(path=w622) -> (name=w623:string)  [unwired: 1 out]
                n322 = local write "V meas"(w627) -> ()
                n323 = local write "I meas"(w626) -> ()
                n324 = Initialize Array(nan ("element"), w632) -> (w631:dbl[])
                n325 = Unbundle By Name(w649) -> ("Wafer Name"=w648:string, "Scribe"=w647:string, "Mask"=w646:string, "Lot"=w645:string)
                n326 = local write "RawData file"(w622) -> ()
                n327 = Bundle("V"=w627, "I"=w626) -> (w630:cluster{"V":dbl[], "I":dbl[]})  [unwired: 1 in]
                n328 = Bundle(w631, w631) -> (w629:cluster{dbl[], dbl[]})  [unwired: 1 in]
                n329 = local write "Test FileName"(w623) -> ()
                n330 = local write "Wafer Name"(w648) -> ()
                n331 = local write "Scribe"(w647) -> ()
                n332 = local write "Mask"(w646) -> ()
                n333 = local write "Lot"(w645) -> ()
                n334 = local write "Selected Data"(w629) -> ()
                n335 = call <vilib>:"Histogram.vi"("X"=w626) -> ("Histogram Graph"=w625:T13)  [unwired: 7 in, 3 out]
                n336 = call <vilib>:"Histogram.vi"("X"=w627) -> ("Histogram Graph"=w624:T13)  [unwired: 7 in, 3 out]
                n337 = Build Array(w630, w629) -> (w628:cluster{"V":dbl[], "I":dbl[]}[])
                n338 = Unbundle By Name(w650) -> ("Device Name"=w644:string, "ActiveArea_um2"=w643:dbl, "MesaArea_um2"=w642:dbl)
                n339 = local write "Vforward hist"(w624) -> ()
                n340 = local write "Idark hist"(w625) -> ()
                n341 = local write "Spec Plot"(w628) -> ()
                n342 = local write "Device Name"(w644) -> ()
                n343 = local write "ActiveArea_um2"(w643) -> ()
                n344 = local write "MesaArea_um2"(w642) -> ()
                n345 = Unbundle By Name(w641) -> ("V set"=w640:dbl, "I compliance"=w639:dbl, "J set"=w638:dbl, "I set"=w637:dbl, "V compliance"=w636:dbl, "Laser Power (mW)"=w634:dbl, "Operator"=w635:string)
                n346 = local write "V set"(w640) -> ()
                n347 = local write "I compliance"(w639) -> ()
                n348 = local write "J set A/cm2"(w638) -> ()
                n349 = local write "I set"(w637) -> ()
                n350 = local write "V compliance"(w636) -> ()
                n351 = local write "Laser Power (mW)"(w634) -> ()
                n352 = local write "Operator"(w635) -> ()
              }
            }
            n353 = Enqueue Element At Opposite End(queue=w618, element="idle", error in (no error)=w617) -> (queue out=w620:refnum<queue>, error out=w619:errorcluster)  [unwired: 1 in, 1 out]
          }
          frame "start fine" {
            n354 = flat-sequence {
              tunnel: [w663] -> w653
              tunnel: w651 -> [w661]
              tunnel: w653 -> [w679]
              frame #0 {
                w664 = u8 0 ("Progress 2")
                n355 = case shown="True" w661 {
                  tunnel: "Mask File Fine" -> [w673 _]
                  tunnel: [w673 w678] -> w659
                  frame False {
                  }
                  frame True {
                    n356 = local read "RawData Save Path"() -> (w675:path)
                    n357 = local read "Wafer Name"() -> (w677:string)
                    n358 = local read "Device Name"() -> (w676:string)
                    n359 = call "Find Latest Fine Mask File.vi"("RawData Save Path"=w675, "Device Name"=w676, "Wafer Name"=w677) -> ("Error Out"=w674:errorcluster, "Mask File Fine"=w678:path)  [unwired: 7 in]
                    n360 = local write "error out"(w674) -> ()
                  }
                }
                n361 = local read "points"() -> (w666:u16)
                n362 = local write "Tab Control"(T12."Fine Test" ("Tab Control")) -> ()
                n363 = Initialize Array(nan ("element"), w666) -> (w668:dbl[])
                n364 = local write "Mask File Fine"(w659) -> ()
                n365 = Bundle(w668, w668) -> (w667:cluster{dbl[], dbl[]})  [unwired: 1 in]
                n366 = call "Device Files v1.vi"("Rows"=1200, "Mask file path"=w659) -> ("size(s)"=w663:i32, "Array of Cell Clusters"=→"Fine Cell Clusters":T3)  [unwired: 6 in, 2 out]
                "Total Device" <- w663
                n367 = local write "Status"("prepare fine test" ("Status")) -> ()
                n368 = local write "Progress 2"(w664) -> ()
                n369 = Initialize Array(w667, w663) -> (→"IV fine linear" →"IV fine log":cluster{dbl[], dbl[]}[])
                "Current Device" <- w664
              }
              frame #1 {
                n370 = for {
                  N: w679 -> [w703]
                  i -> [w704]
                  n371 = Increment(x=w704) -> (x+1=w683:i32)
                  n372 = flat-sequence {
                    tunnel: w704 -> [w710]
                    tunnel: [w718] -> w698
                    tunnel: [w717] -> w697
                    tunnel: [w714] -> w696
                    tunnel: [w713] -> w695
                    tunnel: [w712] -> w694
                    tunnel: [w711] -> w693
                    tunnel: [w710] -> w684
                    tunnel: w698 -> [w733]
                    tunnel: w697 -> [w732]
                    tunnel: w696 -> [w730]
                    tunnel: w695 -> [w729]
                    tunnel: w694 -> [w728]
                    tunnel: w693 -> [w727]
                    tunnel: [w726] -> w692
                    tunnel: [w725] -> w691
                    tunnel: [w724] -> w685
                    tunnel: w684 -> [w724]
                    tunnel: w692 -> [w736]
                    tunnel: w691 -> [w735]
                    tunnel: [w734] -> w686
                    tunnel: w685 -> [w734]
                    tunnel: [w740] -> w687
                    tunnel: w686 -> [w740]
                    tunnel: w687 -> [w770]
                    tunnel: [w760] -> w682
                    tunnel: [w754] -> w681
                    tunnel: [w753] -> w680
                    tunnel: w682 -> [w787]
                    tunnel: w681 -> [w780]
                    tunnel: w680 -> [w779]
                    frame #0 {
                      n373 = local read "Fine Cell Clusters"() -> (w723:T3)
                      n374 = local read "Laser Power (mW)"() -> (w706:dbl)
                      n375 = local read "Prober GPIB"() -> (w719:string)
                      n376 = Index Array(array=w723, index=w710) -> (element=w707:T19)
                      n377 = Unbundle By Name(w707) -> ("Cell Name"=w722:string, "X-coord"=w712:dbl, "Y-coord"=w711:dbl, "Area"=w721:dbl, "Mesa Area"=w720:dbl)
                      n378 = local read "current x"() -> (w716:i32)
                      n379 = local read "current y"() -> (w715:i32)
                      n380 = call "get Area.vi"("Laser"=w706, "Cell Data Cluster"=w707) -> ("Area"=w708:dbl)  [unwired: 9 in]
                      n381 = local read "Parameters Flash 2"() -> (w709:T2)
                      n382 = Bundle By Name(cluster=w709, "Cell Area (cm²)"=w708) -> (w705:T2)
                      n383 = call "EG2001 Move Z Down.vi"("GPIB Address"=w719) -> ("Error Out"=w717:errorcluster, "GPIB Address Out"=w718:string)  [unwired: 9 in]
                      n384 = local write "Parameters Flash"(w705) -> ()
                      n385 = Subtract(x=w712, y=w716) -> (x-y=w714:dbl)
                      n386 = Subtract(x=w711, y=w715) -> (x-y=w713:dbl)
                      n387 = local write "Device Name"(w722) -> ()
                      n388 = local write "ActiveArea_um2"(w721) -> ()
                      n389 = local write "MesaArea_um2"(w720) -> ()
                    }
                    frame #1 {
                      n390 = local write "current x"(w728) -> ()
                      n391 = local write "current y"(w727) -> ()
                      n392 = call "EG2001 Move Machine Step X-Y.vi"("Y"=w729, "Steps/Microns"=enum32{"Steps", "Microns"}."Microns", "X"=w730, "error in (no error)"=w732, "GPIB Address"=w733) -> ("Error Out"=w725:errorcluster, "GPIB Address Out"=w726:string)  [unwired: 5 in]
                    }
                    frame #2 {
                      n393 = call "EG2001 Move Z Up.vi"("error in (no error)"=w735, "GPIB Address"=w736) -> ()  [unwired: 10 out]
                    }
                    frame #3 {
                      n394 = local read "SMU"() -> (w752:refnum<visa-resource-name>)
                      n395 = local read "Sweep Settings"() -> (w751:T8)
                      n396 = local read "Channel"() -> (w749:enum32{"Channel A", "Channel B"})
                      n397 = local read "V start"() -> (w747:dbl)
                      n398 = local read "V end"() -> (w748:dbl)
                      n399 = local read "points"() -> (w746:u16)
                      n400 = local read "NPLC"() -> (w745:dbl)
                      n401 = local read "I compliance"() -> (w744:dbl)
                      n402 = local read "sweep delay ms"() -> (w743:dbl)
                      n403 = local read "Device Name"() -> (w738:string)
                      n404 = local read "Wafer Info Flash 2"() -> (w739:T1)
                      n405 = Bundle By Name(cluster=w739, "Cell Name"=w738) -> (w737:T1)
                      n406 = local write "Wafer Info Flash"(w737) -> ()
                      n407 = Bundle By Name(cluster=w751, "Channel"=w749, "Vstart"=w747, "Vend"=w748, "# of points"=w746, "NPLC"=w745, "I compliance"=w744, "Delay ms"=w743) -> (w750:T8)
                      n408 = call "K2602 Vsweep.vi"("Settings"=w750, "SMU"=w752) -> ("V"=w741:dbl[], "I"=w742:dbl[])  [unwired: 7 in, 1 out]
                      n409 = local write "I fine"(w742) -> ()
                      n410 = local write "V fine"(w741) -> ()
                    }
                    frame #4 {
                      n411 = local read "V fine"() -> (w759:dbl[])
                      n412 = local read "I fine"() -> (w766:dbl[])
                      n413 = local read "IV fine linear"() -> (w773:cluster{dbl[], dbl[]}[])
                      n414 = local read "IV fine log"() -> (w768:cluster{dbl[], dbl[]}[])
                      n415 = local read "Wafer Name"() -> (w763:string)
                      n416 = local read "Operator"() -> (w762:string)
                      n417 = local read "Device Name"() -> (w761:string)
                      n418 = Get Date/Time In Seconds() -> (seconds since 1Jan1904=w753:timestamp)
                      n419 = local read "current x"() -> (w756:i32)
                      n420 = local read "current y"() -> (w755:i32)
                      n421 = Absolute Value(x=w766) -> (abs(x)=w767:dbl[])
                      n422 = Bundle("V fine"=w759, "I fine"=w766) -> (w771:cluster{"V fine":dbl[], "I fine":dbl[]})  [unwired: 1 in]
                      n423 = To Double Precision Float(number=w756) -> (double precision float=w758:dbl)
                      n424 = To Double Precision Float(number=w755) -> (double precision float=w757:dbl)
                      n425 = Bundle("V fine"=w759, w767) -> (w765:cluster{"V fine":dbl[], dbl[]})  [unwired: 1 in]
                      n426 = Replace Array Subset(array=w768, new element=w765, index=w770) -> (w769:cluster{dbl[], dbl[]}[])
                      n427 = local write "IV fine log"(w769) -> ()
                      n428 = Replace Array Subset(array=w773, new element=w771, index=w770) -> (w772:cluster{dbl[], dbl[]}[])
                      n429 = local write "IV fine linear"(w772) -> ()
                      n430 = Bundle(w758, w757) -> (w754:cluster{dbl, dbl})  [unwired: 1 in]
                      n431 = call "get Flash FileName .vi"("Time"=w753, "Device Name"=w761, "Operator"=w762, "Wafer Name"=w763, "FineTest save path"="FineTest save path") -> ("appended path"=w760:path)  [unwired: 6 in]
                    }
                    frame #5 {
                      n432 = local read "Parameters Flash"() -> (w782:T2)
                      n433 = local read "Wafer Info Flash"() -> (w781:T1)
                      n434 = local read "I fine"() -> (w785:dbl[])
                      n435 = local read "V fine"() -> (w784:dbl[])
                      n436 = local read "Mask"() -> (w786:string)
                      n437 = Get Date/Time String(seconds (now)=w779, want seconds? (F)=TRUE) -> (date string=w778:string, time string=w775:string)  [unwired: 1 in]
                      n438 = call <vilib>:"Space Constant.vi"() -> ("String"=w774:string)
                      n439 = Concatenate Strings(w778, w774, w775) -> (w776:string)
                      n440 = Build Array(w785, w784) -> (w783:dbl[][])
                      n441 = call "WriteFlashFile.vi"("file path (dialog if empty)"=w787, "Mask Name"=w786, "IV array"=w783, "Date/Time String"=w776, "Parameters"=w782, "Coords"=w780, "Wafer Info"=w781) -> ()  [unwired: 8 in, 1 out]
                    }
                  }
                  n442 = Divide(x=w683, y=w703) -> (x/y=w702:dbl)
                  n443 = Multiply(x=100.0, y=w702) -> (x*y=w700:dbl)
                  n444 = To Unsigned Byte Integer(number=w700) -> (unsigned 8bit integer=w699:u8)
                  n445 = local write "Progress 2"(w699) -> ()
                  n446 = local write "Current Device"(w683) -> ()
                  n447 = Number To Decimal String(number=w683) -> (decimal integer string=w689:string)  [unwired: 1 in]
                  n448 = Concatenate Strings("IV test for die number: " ("string"), w689) -> (w688:string)
                  n449 = local write "Status"(w688) -> ()
                }
              }
              frame #2 {
                w792 = -1 ("x")
                n450 = local read "current x"() -> (w794:i32)
                n451 = local read "current y"() -> (w793:i32)
                n452 = local read "Prober GPIB"() -> (w796:string)
                n453 = call "EG2001 Move Z Down.vi"("GPIB Address"=w796) -> ("Error Out"=w795:errorcluster, "GPIB Address Out"=w797:string)  [unwired: 9 in]
                n454 = Multiply(x=w792, y=w794) -> (x*y=w791:i32)
                n455 = Multiply(x=w793, y=w792) -> (x*y=w790:i32)
                n456 = call "EG2001 Move Machine Step X-Y.vi"("Flip X Coordinates?"=FALSE, "Y"=w790, "Steps/Microns"=enum32{"Steps", "Microns"}."Microns", "X"=w791, "error in (no error)"=w795, "GPIB Address"=w797) -> ()  [unwired: 4 in, 2 out]
              }
              frame #3 {
                w798 = 0 ("current x")
                n457 = local write "current x"(w798) -> ()
                n458 = local write "current y"(w798) -> ()
              }
            }
            n459 = Enqueue Element At Opposite End(queue=w656, element="idle", error in (no error)=w655) -> (queue out=w658:refnum<queue>, error out=w657:errorcluster)  [unwired: 1 in, 1 out]
          }
          frame "raw mask updated" {
            n460 = Two Button Dialog(message="Wold you like to update the Manual mask?", 1:"No" ("F button name (\"Cancel\")"), 2:"Yes" ("T button name (\"OK\")")) -> (T button?=w799:bool)
            n461 = case shown="True" w799 {
              frame False {
              }
              frame True {
                n462 = local read "Mask File Raw"() -> (w809:path)
                n463 = local write "Mask File Manual"(w809) -> ()
              }
            }
            n464 = Enqueue Element At Opposite End(queue=w806, element="idle", error in (no error)=w805) -> (queue out=w808:refnum<queue>, error out=w807:errorcluster)  [unwired: 1 in, 1 out]
          }
          frame "mask manual update" {
            n465 = Two Button Dialog(message="Would you like update mask file for raw test?", 1:"No" ("F button name (\"Cancel\")"), 2:"Yes" ("T button name (\"OK\")")) -> (T button?=w810:bool)
            n466 = case shown="True" w810 {
              frame False {
              }
              frame True {
                n467 = local read "Mask File Manual"() -> (w820:path)
                n468 = local write "Mask File Raw"(w820) -> ()
              }
            }
            n469 = Enqueue Element At Opposite End(queue=w817, element="idle", error in (no error)=w816) -> (queue out=w819:refnum<queue>, error out=w818:errorcluster)  [unwired: 1 in, 1 out]
          }
          frame "refresh device names" {
            n470 = call "getDB unique Device.vi"("Mask"="Mask Name") -> ("NameList"=w821:string[])  [unwired: 9 in, 1 out]
            "NameList" <- w821
            n471 = property on="Available Device Name" class="CmbBox"("Strings[]"=w821) -> ()  [unwired: 2 in, 2 out]
            n472 = Enqueue Element At Opposite End(queue=w826, element="idle", error in (no error)=w825) -> (queue out=w828:refnum<queue>, error out=w827:errorcluster)  [unwired: 1 in, 1 out]
          }
          frame "add to list" {
            n473 = local read "Available Device Name"() -> (w830:string)
            n474 = property on="Test List" class="LstBox (strict)"() -> ("Item Names"=w831:string[])  [unwired: 2 in, 2 out]
            n475 = Build Array (concatenate)(w831, w830) -> (w829:string[])
            n476 = property on="Test List" class="LstBox (strict)"("Item Names"=w829) -> ()  [unwired: 2 in, 2 out]
            n477 = Enqueue Element At Opposite End(queue=w835, element="idle", error in (no error)=w833) -> (queue out=w837:refnum<queue>, error out=w836:errorcluster)  [unwired: 1 in, 1 out]
          }
          frame "remove from list" {
            n478 = local read "Test List"() -> (w838:i32)
            n479 = property on="Test List" class="LstBox (strict)"() -> ("Item Names"=w840:string[])  [unwired: 2 in, 2 out]
            n480 = Delete From Array(array=w840, index=w838) -> (array with subset deleted=w839:string[])  [unwired: 1 in, 1 out]
            n481 = property on="Test List" class="LstBox (strict)"("Item Names"=w839) -> ()  [unwired: 2 in, 2 out]
            n482 = Enqueue Element At Opposite End(queue=w842, element="idle", error in (no error)=w841) -> (queue out=w844:refnum<queue>, error out=w843:errorcluster)  [unwired: 1 in, 1 out]
          }
          frame "clear list" {
            n483 = property on="Test List" class="LstBox (strict)"("Item Names"=string[] []) -> ()  [unwired: 2 in, 2 out]
            n484 = Enqueue Element(queue=w851, element="idle", error in (no error)=w849) -> (queue out=w853:refnum<queue>, error out=w852:errorcluster)  [unwired: 1 in, 1 out]
          }
          frame "pick device" {
            n485 = flat-sequence {
              frame #0 {
                n486 = property on="Test List" class="LstBox (strict)"() -> ("Item Names"=w864:string[])  [unwired: 2 in, 2 out]
                n487 = local read "Counter"() -> (w863:i32)
                n488 = Index Array(array=w864, index=w863) -> (element=w860:string)
                n489 = local read "Mask File all"() -> (w862:path)
                n490 = local write "Device Name"(w860) -> ()
                n491 = call "Mask file select device.vi"("Device"=w860, "MaskFile"=w862) -> ("RawMask"=w861:path)  [unwired: 9 in]
                n492 = local write "Mask File Raw"(w861) -> ()
              }
              frame #1 {
                n493 = local read "Counter"() -> (w866:i32)
                n494 = Increment(x=w866) -> (x+1=w865:i32)
                n495 = local write "Counter"(w865) -> ()
              }
              frame #2 {
                n496 = local read "Counter"() -> (w870:i32)
                n497 = property on="Test List" class="LstBox (strict)"() -> ("Item Names"=w869:string[])  [unwired: 2 in, 2 out]
                n498 = Array Size(array=w869) -> (size(s)=w868:i32)
                n499 = Equal?(x=w870, y=w868) -> (x = y?=w867:bool)
                n500 = case shown="False" w867 {
                  frame False {
                  }
                  frame True {
                    n501 = local write "Counter"(0 ("Counter")) -> ()
                  }
                }
              }
            }
            n502 = Enqueue Element(queue=w859, element="idle", error in (no error)=w857) -> (queue out=w858:refnum<queue>, error out=w856:errorcluster)  [unwired: 1 in, 1 out]
          }
        }
      }
      n503 = while {
        shift-right: [w22] -> w18
        shift-left: w17 -> [w23]
        shift-right: [w20] -> w9
        shift-left: w16 -> [w21]
        stop <- w24 stop-if-true
        n504 = event shown="[21] \"Start auto\": Value Change" {
          selector: _ -> [_ _ _ _ _ _ _ _ _ _ _ _ _ _ _ _ _ _ _ _ _ _]
          dyn-events: _ -> [_ _ _ _ _ _ _ _ _ _ _ _ _ _ _ _ _ _ _ _ _ _]
          timeout: -1 -> [_ _ _ _ _ _ _ _ _ _ _ _ _ _ _ _ _ _ _ _ _ _]
          tunnel: [_ TRUE _ _ _ _ _ _ FALSE _ _ _ _ _ _ _ _ _ _ _ _ _] -> w24
          tunnel: w23 -> [w28 w40 w50 w55 w60 w64 w68 w75 w81 w86 w91 w96 w101 w106 w111 w116 w121 w126 w131 w136 w141 w146]
          tunnel: [_ w44 w49 w54 w59 w62 w67 _ w80 w85 w90 w94 w99 w104 w109 w114 w119 w124 w129 w135 w139 w145] -> w22
          tunnel: w21 -> [w27 w43 w48 w53 w58 w63 w69 w74 w78 w84 w89 w95 w100 w105 w110 w115 w120 w125 w130 w134 w140 w144]
          tunnel: [w26 w42 w47 w52 _ w61 w66 _ w79 w83 w88 w93 w98 w103 w108 w113 w118 w123 w128 w133 w138 w143] -> w20
          tunnel: [_ _ _ _ _ _ _ w73 _ _ _ _ _ _ _ _ _ _ _ _ _ _] -> _
          tunnel: [_ _ _ _ _ _ _ w72 _ _ _ _ _ _ _ _ _ _ _ _ _ _] -> _
          tunnel: [w25 _ _ _ _ _ _ _ _ _ _ _ _ _ _ _ _ _ _ _ _ _] -> _
          tunnel: [_ _ _ _ w57 _ _ _ _ _ _ _ _ _ _ _ _ _ _ _ _ _] -> _
          event Timeout {
            n505 = event-data() -> ()  [unwired: 1 in, 2 out]
            n506 = First Call?() -> (First Call?: T/F=w29:bool)
            n507 = case shown="True" w29 {
              tunnel: w27 -> [w32 w38]
              tunnel: w28 -> [w34 w39]
              tunnel: [w31 w37] -> w26
              tunnel: [w33 w36] -> w25
              frame False {
                n508 = Enqueue Element(queue=w34, element="idle", error in (no error)=w32) -> (queue out=w33:refnum<queue>, error out=w31:errorcluster)  [unwired: 1 in, 1 out]
              }
              frame True {
                n509 = Enqueue Element(queue=w39, element="load file manual", error in (no error)=w38) -> (queue out=w36:refnum<queue>, error out=w37:errorcluster)  [unwired: 1 in, 1 out]
              }
            }
          }
          event "stop": Value Change {
            n510 = event-data() -> ()  [unwired: 1 in, 5 out]
            n511 = Enqueue Element(queue=w40, element="stop", error in (no error)=w43) -> (queue out=w44:refnum<queue>, error out=w42:errorcluster)  [unwired: 1 in, 1 out]
          }
          event "StartRaw": Value Change {
            n512 = event-data() -> ()  [unwired: 1 in, 5 out]
            n513 = Enqueue Element(queue=w50, element="start raw", error in (no error)=w48) -> (queue out=w49:refnum<queue>, error out=w47:errorcluster)  [unwired: 1 in, 1 out]
          }
          event "load file": Value Change {
            n514 = event-data() -> ()  [unwired: 1 in, 5 out]
            n515 = Enqueue Element(queue=w55, element="load file manual", error in (no error)=w53) -> (queue out=w54:refnum<queue>, error out=w52:errorcluster)  [unwired: 1 in, 1 out]
          }
          event "Die Number": Value Change {
            n516 = event-data() -> ()  [unwired: 1 in, 5 out]
            n517 = Enqueue Element(queue=w60, element="Die number picked", error in (no error)=w58) -> (queue out=w59:refnum<queue>, error out=w57:errorcluster)  [unwired: 1 in, 1 out]
          }
          event "Move to": Value Change {
            n518 = event-data() -> ()  [unwired: 1 in, 5 out]
            n519 = Enqueue Element(queue=w64, element="moveto", error in (no error)=w63) -> (queue out=w62:refnum<queue>, error out=w61:errorcluster)  [unwired: 1 in, 1 out]
          }
          event "Manual_Test": Value Change {
            n520 = event-data() -> ()  [unwired: 1 in, 5 out]
            n521 = Enqueue Element(queue=w68, element="manual test", error in (no error)=w69) -> (queue out=w67:refnum<queue>, error out=w66:errorcluster)  [unwired: 1 in, 1 out]
          }
          event "J set A/cm2": Value Change {
            n522 = event-data() -> ()  [unwired: 1 in, 5 out]
            n523 = Enqueue Element(queue=w75, element="Jset change", error in (no error)=w74) -> (queue out=w73:refnum<queue>, error out=w72:errorcluster)  [unwired: 1 in, 1 out]
          }
          event "Reset xy": Value Change {
            n524 = event-data() -> ()  [unwired: 1 in, 5 out]
            n525 = Enqueue Element(queue=w81, element="reset xy", error in (no error)=w78) -> (queue out=w80:refnum<queue>, error out=w79:errorcluster)  [unwired: 1 in, 1 out]
          }
          event "Reset 1st die": Value Change {
            n526 = event-data() -> ()  [unwired: 1 in, 5 out]
            n527 = Enqueue Element(queue=w86, element="reset to 1st die", error in (no error)=w84) -> (queue out=w85:refnum<queue>, error out=w83:errorcluster)  [unwired: 1 in, 1 out]
          }
          event "Manual IV settting": Value Change {
            n528 = event-data() -> ()  [unwired: 1 in, 5 out]
            n529 = Enqueue Element(queue=w91, element="change plot", error in (no error)=w89) -> (queue out=w90:refnum<queue>, error out=w88:errorcluster)  [unwired: 1 in, 1 out]
          }
          event "update wafer": Value Change {
            n530 = event-data() -> ()  [unwired: 1 in, 5 out]
            n531 = Enqueue Element(queue=w96, element="update wafer", error in (no error)=w95) -> (queue out=w94:refnum<queue>, error out=w93:errorcluster)  [unwired: 1 in, 1 out]
          }
          event "Select": Value Change {
            n532 = event-data() -> ()  [unwired: 1 in, 5 out]
            n533 = Enqueue Element(queue=w101, element="select", error in (no error)=w100) -> (queue out=w99:refnum<queue>, error out=w98:errorcluster)  [unwired: 1 in, 1 out]
          }
          event "StartFine": Value Change {
            n534 = event-data() -> ()  [unwired: 1 in, 5 out]
            n535 = Enqueue Element(queue=w106, element="start fine", error in (no error)=w105) -> (queue out=w104:refnum<queue>, error out=w103:errorcluster)  [unwired: 1 in, 1 out]
          }
          event "Mask File Raw": Value Change {
            n536 = event-data() -> ()  [unwired: 1 in, 5 out]
            n537 = Enqueue Element(queue=w111, element="raw mask updated", error in (no error)=w110) -> (queue out=w109:refnum<queue>, error out=w108:errorcluster)  [unwired: 1 in, 1 out]
          }
          event "Mask File Manual": Value Change {
            n538 = event-data() -> ()  [unwired: 1 in, 5 out]
            n539 = Enqueue Element(queue=w116, element="mask manual update", error in (no error)=w115) -> (queue out=w114:refnum<queue>, error out=w113:errorcluster)  [unwired: 1 in, 1 out]
          }
          event "Load raw": Value Change {
            n540 = event-data() -> ()  [unwired: 1 in, 5 out]
            n541 = Enqueue Element(queue=w121, element="load raw data", error in (no error)=w120) -> (queue out=w119:refnum<queue>, error out=w118:errorcluster)  [unwired: 1 in, 1 out]
          }
          event "Refresh Device": Value Change {
            n542 = event-data() -> ()  [unwired: 1 in, 5 out]
            n543 = Enqueue Element(queue=w126, element="refresh device names", error in (no error)=w125) -> (queue out=w124:refnum<queue>, error out=w123:errorcluster)  [unwired: 1 in, 1 out]
          }
          event "Add to list": Value Change {
            n544 = event-data() -> ()  [unwired: 1 in, 5 out]
            n545 = Enqueue Element(queue=w131, element="add to list", error in (no error)=w130) -> (queue out=w129:refnum<queue>, error out=w128:errorcluster)  [unwired: 1 in, 1 out]
          }
          event "Remove from List": Value Change {
            n546 = event-data() -> ()  [unwired: 1 in, 5 out]
            n547 = Enqueue Element(queue=w136, element="remove from list", error in (no error)=w134) -> (queue out=w135:refnum<queue>, error out=w133:errorcluster)  [unwired: 1 in, 1 out]
          }
          event "Clear List": Value Change {
            n548 = event-data() -> ()  [unwired: 1 in, 5 out]
            n549 = Enqueue Element(queue=w141, element="clear list", error in (no error)=w140) -> (queue out=w139:refnum<queue>, error out=w138:errorcluster)  [unwired: 1 in, 1 out]
          }
          event "Start auto": Value Change {
            n550 = event-data() -> ()  [unwired: 1 in, 1 out]
            n551 = property on="Test List" class="LstBox (strict)"() -> ("Item Names"=w142:string[])  [unwired: 2 in, 2 out]
            n552 = for {
              shift-right: [w149] -> w143
              shift-left: w144 -> [w155]
              shift-right: [w150] -> w145
              shift-left: w146 -> [w156]
              tunnel: w142 -> [_] mode=indexing
              n553 = local read "Laser Power (mW)"() -> (w148:dbl)
              n554 = Enqueue Element(queue=w156, element="pick device", error in (no error)=w155) -> (queue out=w154:refnum<queue>, error out=w153:errorcluster)  [unwired: 1 in, 1 out]
              n555 = Greater Than 0?(x=w148) -> (x > 0?=w147:bool)
              n556 = case shown="True" w147 {
                tunnel: w154 -> [w162 w167]
                tunnel: w153 -> [w161 w168]
                tunnel: [w160 w167] -> w152
                tunnel: [w159 w168] -> w151
                frame False {
                  n557 = Enqueue Element(queue=w162, element="start raw", error in (no error)=w161) -> (queue out=w165:refnum<queue>, error out=w166:errorcluster)  [unwired: 1 in, 1 out]
                  n558 = Enqueue Element(queue=w165, element="select", error in (no error)=w166) -> (queue out=w160:refnum<queue>, error out=w159:errorcluster)  [unwired: 1 in, 1 out]
                }
                frame True {
                }
              }
              n559 = Enqueue Element(queue=w152, element="start fine", error in (no error)=w151) -> (queue out=w150:refnum<queue>, error out=w149:errorcluster)  [unwired: 1 in, 1 out]
            }
          }
        }
      }
      n560 = Release Queue(queue=w18, force destroy? (F)=TRUE, error in (no error)=w9) -> (error out=→"error out":errorcluster)  [unwired: 2 out]
    }
  }
